vi "RF Paths Calibration Tool.vi"() -> ()   [LabVIEW 2015]
uses:
  <instrlib>/niRFSG/niRFSG.llb/niRFSG Ref Clock Sources.ctl
  <vilib>/Utility/file.llb/Read From Spreadsheet File (DBL).vi
  <vilib>/Utility/file.llb/Write To Spreadsheet File (DBL).vi
panel:
  out "Frequency (Hz)":dbl format="%.3p"
  out "Corrected Pwr (dBm)":dbl format="%.3g"
  in  "SG_Type":enum32{"ESG/PSG", "RFSG"}(tab)
  in  "Power Level Ref-ESG(dBm)":dbl caption="Power Level (dBm)" format="%.2f"
  in  "ALC":bool=TRUE
  in  "ALC BW":bool=TRUE
  in  "Pwr Srch":bool
  in  "Freq Mode":bool=TRUE
  in  "SigGen (ESG)":refnum<visa-resource-name>
  in  "Power Level - RFSG(dBm)":dbl caption="Power Level (dBm)" format="%.2f"
  in  "SigGen (RFSG)":refnum<k15>
  in  "Loop Delay(ms)":i32=100
  in  "Secure Display":bool
  in  "Config Save":bool
  in  "Start":bool
  in  "Stop":bool
  in  "Help":bool
  out "main_queue":refnum<user-event>
  in  "Export Plots to Excel?":bool
  in  "PM Type":T1(tab)=enum."U2000 USB [PM2]"
  in  "Measuring Function":i32(ring) items=["Single", "Single Relative", "Difference", "Difference Relative", "Ratio", "Ratio Relative"]
  in  "Channel":i32(ring) items=["A", "B"]
  in  "Resolution":i32=3
  in  "Avg Count":i32=3
  in  "PM State":bool
  in  "Measurement Speed":i32(ring)=2 items=["Normal", "Double", "Fast"]
  in  "Sensor 1 Channel":i32(ring) items=["Channel A", "Channel B"]
  in  "Sensor 2 Channel":i32(ring) items=["Channel A", "Channel B"]
  in  "Auto Clear":i32(ring) items=["Off", "On", "ONCE"]
  in  "EPM GPIB ALIAS":refnum<visa-resource-name>
  in  "Units":i32(ring) items=["dBm", "W"]
  in  "Trigger Level (dBm)":dbl
  in  "Averaging Count":i32=3 min=1 max=100 step=1
  in  "Trigger Source":i32(ring)=3 items=["Bus", "External", "Hold", "Immediate", "Internal A"]
  in  "Trigger Slope":u16(ring) items=["Positive", "Negative"]
  in  "Enable Averaging":bool
  in  "U2000 GPIB ALIAS":refnum<visa-resource-name>
  in  "Atten (dB)":dbl=20.0
  in  "Auto Atten":bool
  in  "Averaging":bool=TRUE
  in  "Auto Align":bool=TRUE
  in  "Zero Span":bool=TRUE
  in  "Avg":i32=10
  in  "Ref Lvl (dBm)":dbl=10.0 min=-100.0 max=30.0 step=0.1
  in  "SpecAn Mode":enum32{"Manual", "Auto"}(tab)
  in  "VBW (Hz)":i32=300000 format="%.0p"
  in  "RBW (Hz)":i32=100000 format="%.0p"
  in  "Span (Hz)":dbl=100000.0 format="%#_13p"
  in  "PSA E4440A GPIB":refnum<visa-resource-name>
  out "Status":string
  out "Path Loss":cluster{dbl[]}[](graph)
  in  "Tab Control":enum32{"Arbitrary", "Lookup Table"}(tab)=enum."Lookup Table"
  in  "Intervals (Hz)":dbl=1000000.0 min=100000.0 max=1000000000.0 step=100000.0 format="%.3p"
  in  "Stop F (Hz)":dbl=6000000000.0 min=1000000.0 max=18000000000.0 step=1000000.0 format="%.3p"
  in  "Start F (Hz)":dbl=10000000.0 min=1000000.0 max=18000000000.0 step=1000000.0 format="%.3p"
  in  "file path (dialog if empty)":path
  out "Normalization Active":bool
  in  "Normalization Files":path[](array[path])
  out "Error Out":errorcluster {"code" format="%.0x"}
  # "rev: 3.0.1"
  # "CW/Signal Generator Configuration"
  # "CW"
  # "FIX"
  # "RBW/VBW Settings\nNot  Required"
  # "Measuring Device Configuration [Select Type]"
  # "Frequency Sweep Parameters"
  # "RF Paths Calibration Tool"
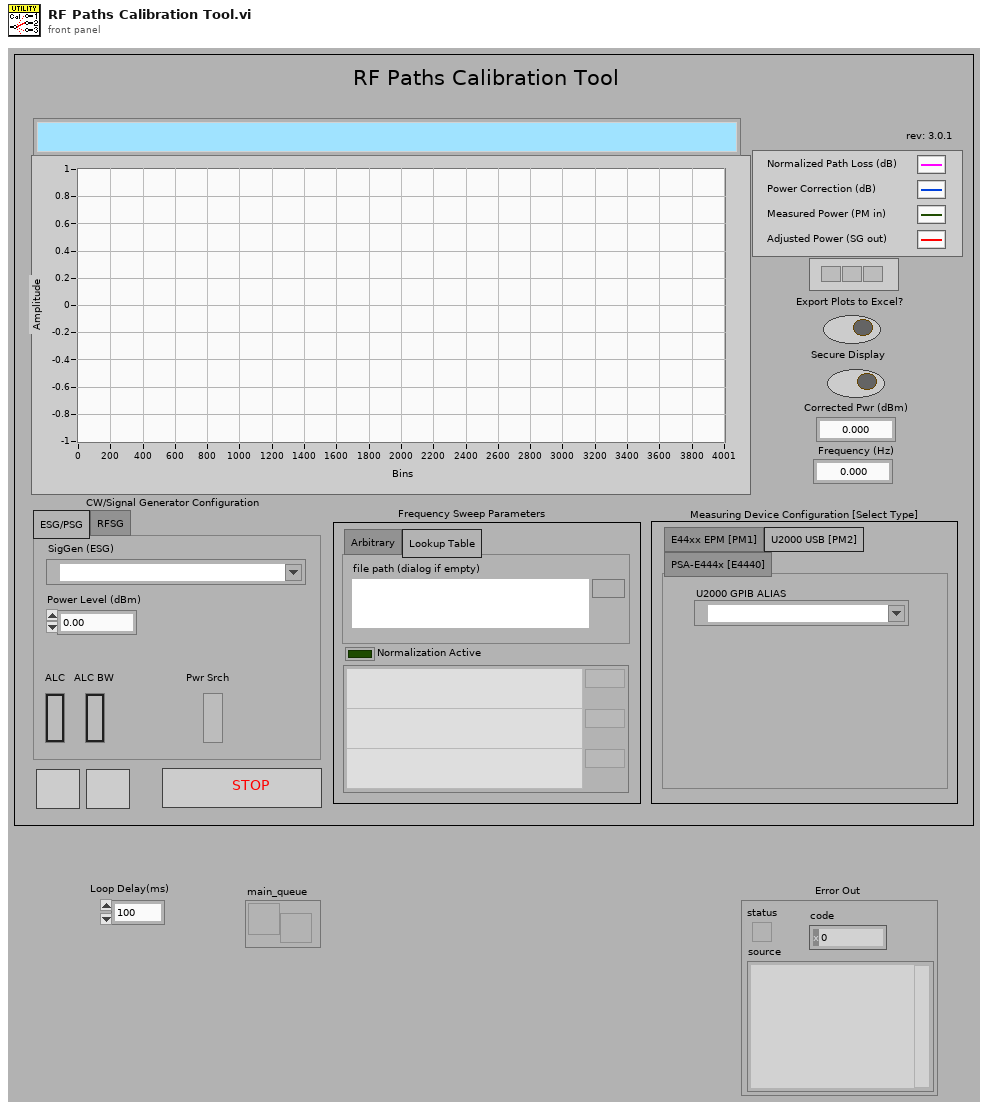
[diagram p1: front panel]
types:
  T1 = enum32{"E44xx EPM [PM1]", "U2000 USB [PM2]", "PSA-E444x [E4440]"}
  T2 = enum32{"invalid app kind", "Development System", "Run Time System", "Student Edition", "Embedded LabVIEW", "Evaluation", "Custom"}
  T3 = enum32{"Invalid", "Standard", "Closed", "Hidden", "Minimized", "Maximized"}
  T4 = typedef "niRFSG Ref Clock Sources.ctl" = string
  T5 = cluster{"INI Path":path, "PSA E4440A GPIB":refnum<visa-resource-name>, "EPM GPIB ALIAS":refnum<visa-resource-name>, "U2000 GPIB ALIAS":refnum<visa-resource-name>, "SigGen (ESG)":refnum<visa-resource-name>, "SigGen (RFSG)":refnum<k15>, "Power Level Ref-ESG(dBm)":dbl, "Power Level - RFSG(dBm)":dbl, "Initial Cal Freq":dbl, "Span (Hz)":dbl, "Cal Freqs":dbl[], "Input Path Loss":dbl[], "ALC":bool, "PM State":bool, "Freq Mode":bool, "Zero Span":bool, "SG_Type":enum32{"ESG/PSG", "RFSG"}, "PM Type":enum32{"E44xx EPM [PM1]", "U2000 USB [PM2]", "PSA-E444x [E4440]"}, "Channel":i32, "Avg Count":i32, "Measurement Speed":i32, "Measuring Function":i32, "Sensor 1 Channel":i32, "Sensor 2 Channel":i32, "Unit (0: dBm)":i32, "Rows":i32, "Normalization Files":path[], "Path Loss":cluster{dbl[]}[], "Input parameters":cluster{"Channel (1)":i32, "Avg Count":i32, "Correction Frequency":dbl, "Timeout":i32, "Reset Device":bool, "ID Query":bool, "Resource Name":string, "Ref Level (dB)":dbl}, "Status":string}
  T6 = cluster{"Core":cluster{"Current VI Reference":refnum<vi>, "Close Panel on Exit?":bool}, "Your Boolean data":bool, "Your string data":string}
  T7 = cluster{"Current VI Reference":refnum<vi>, "Close Panel on Exit?":bool}
  T8 = cluster{"Channel (1)":i32, "Avg Count":i32, "Correction Frequency":dbl, "Timeout":i32, "Reset Device":bool, "ID Query":bool, "Resource Name":string, "Ref Level (dB)":dbl}
  T9 = enum8{"Enabled", "Disabled", "Disabled and Grayed Out"}
  T10 = enum16{"Left Button", "Center Button", "Right Button", "Window Close"}
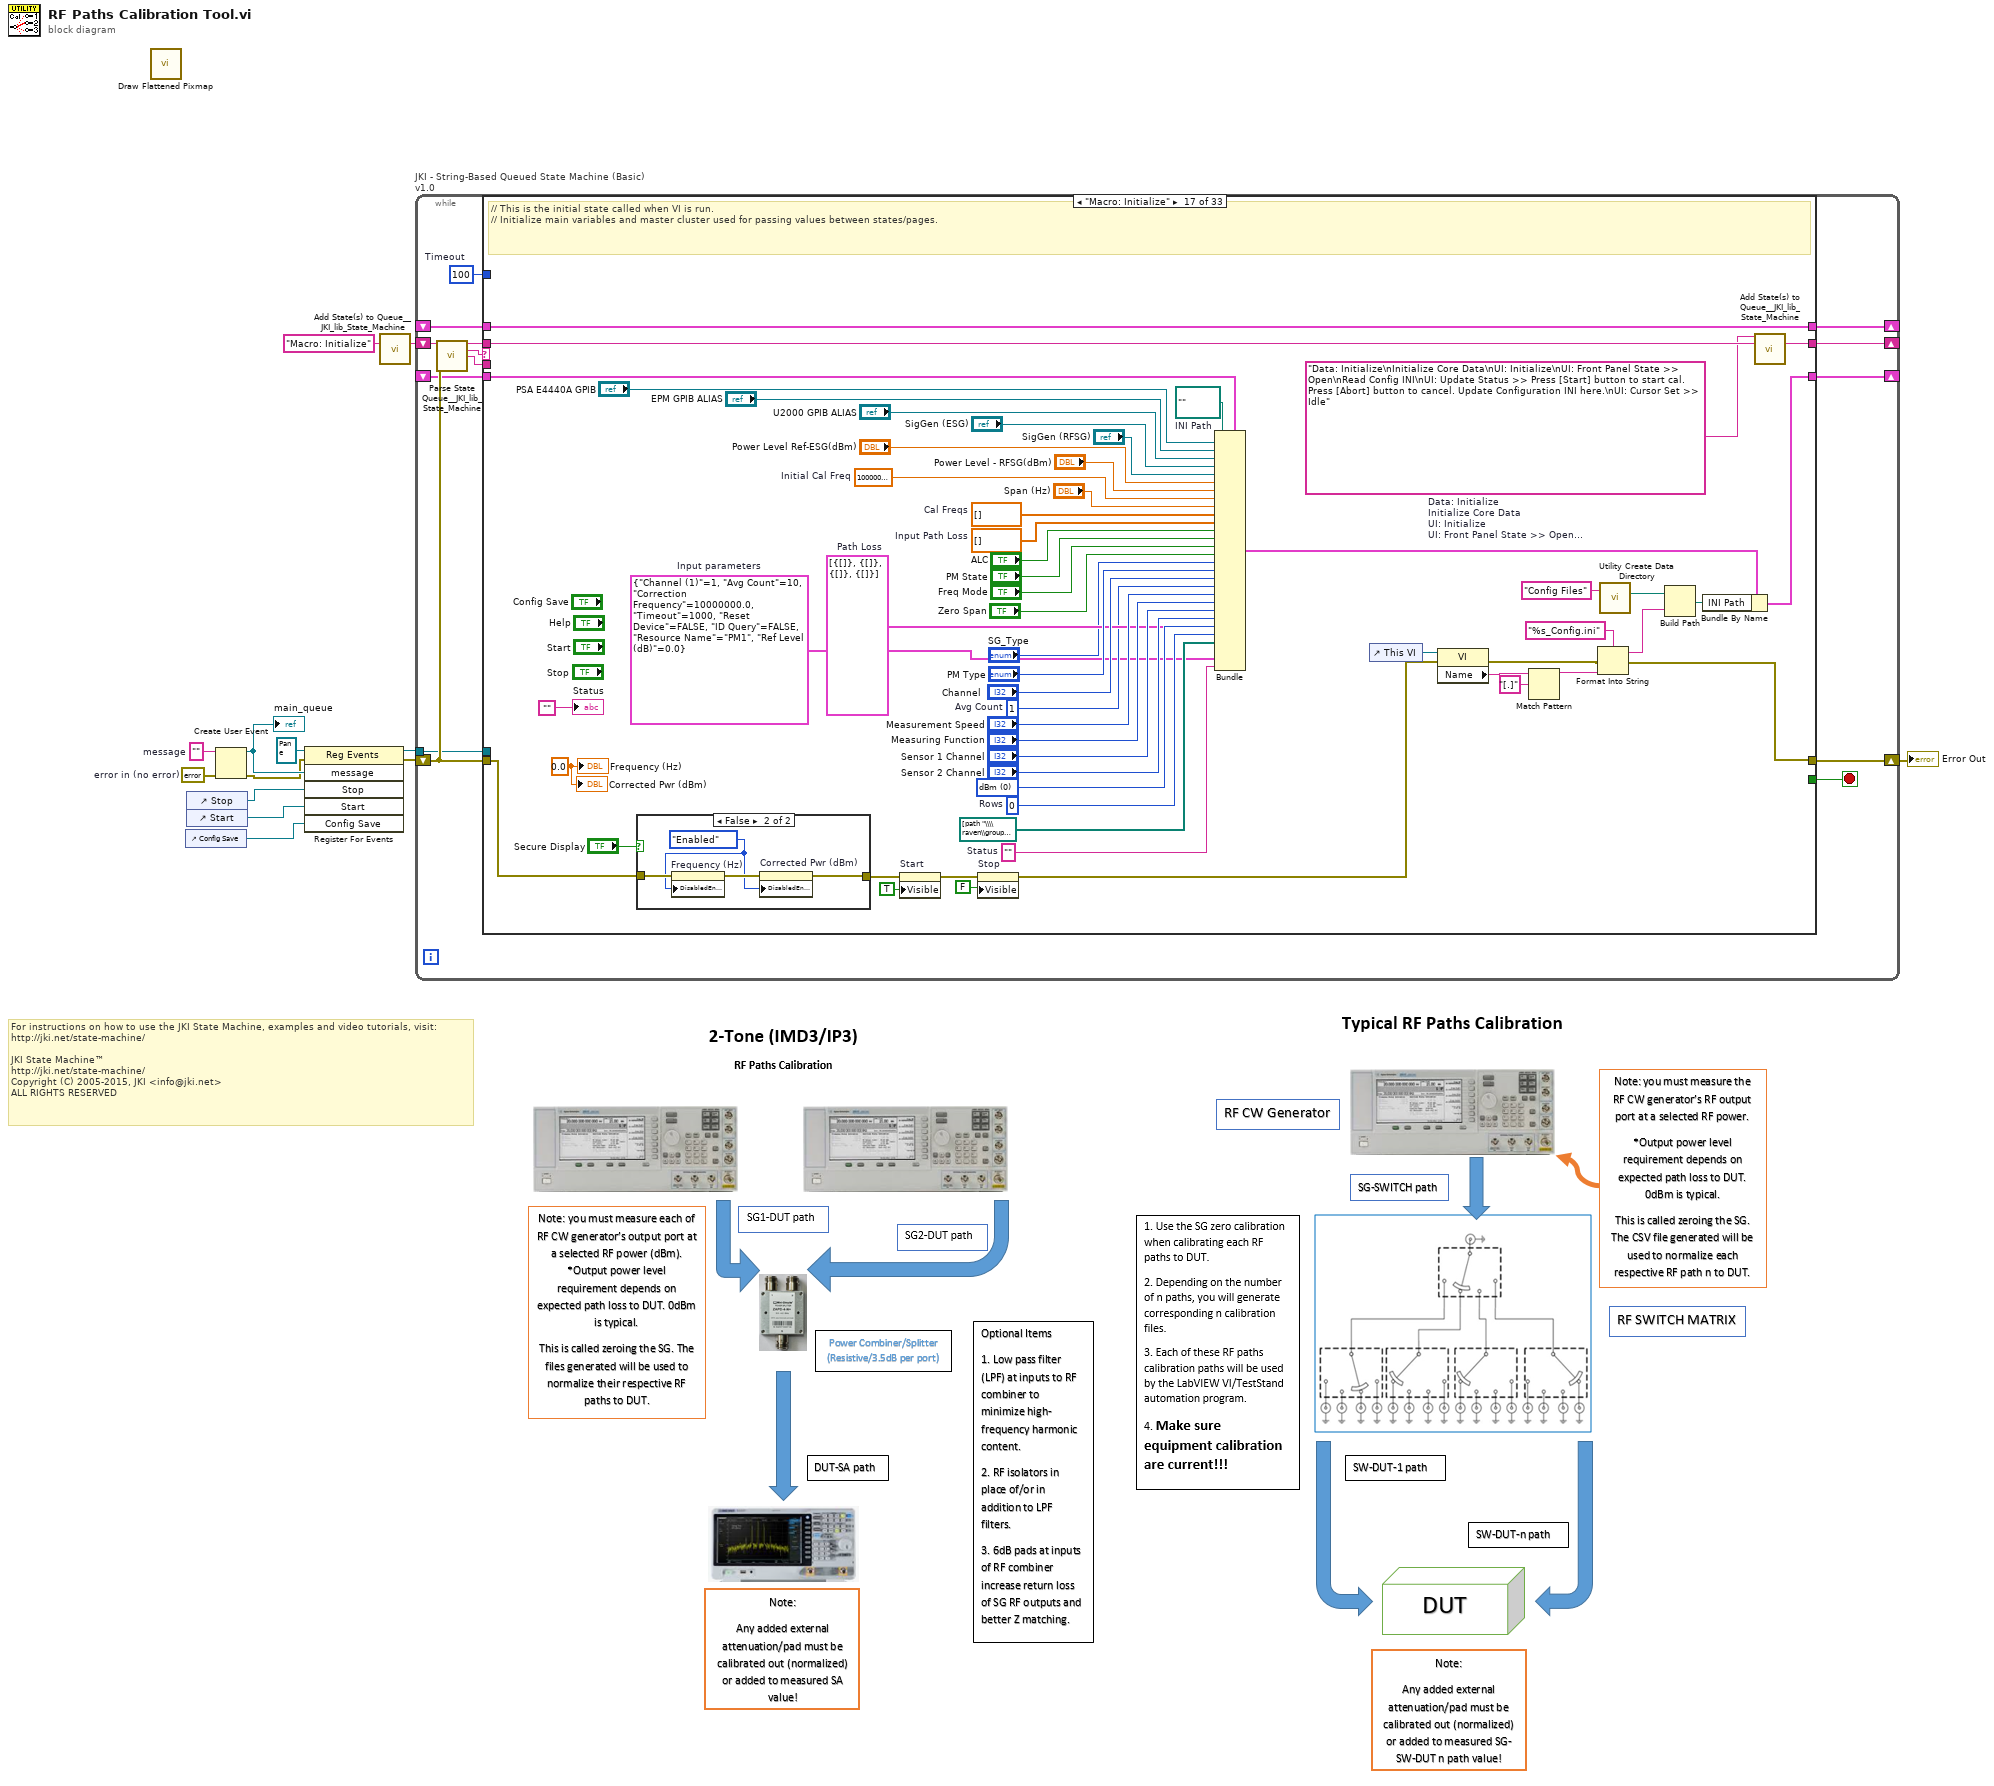
[diagram p0: block diagram]
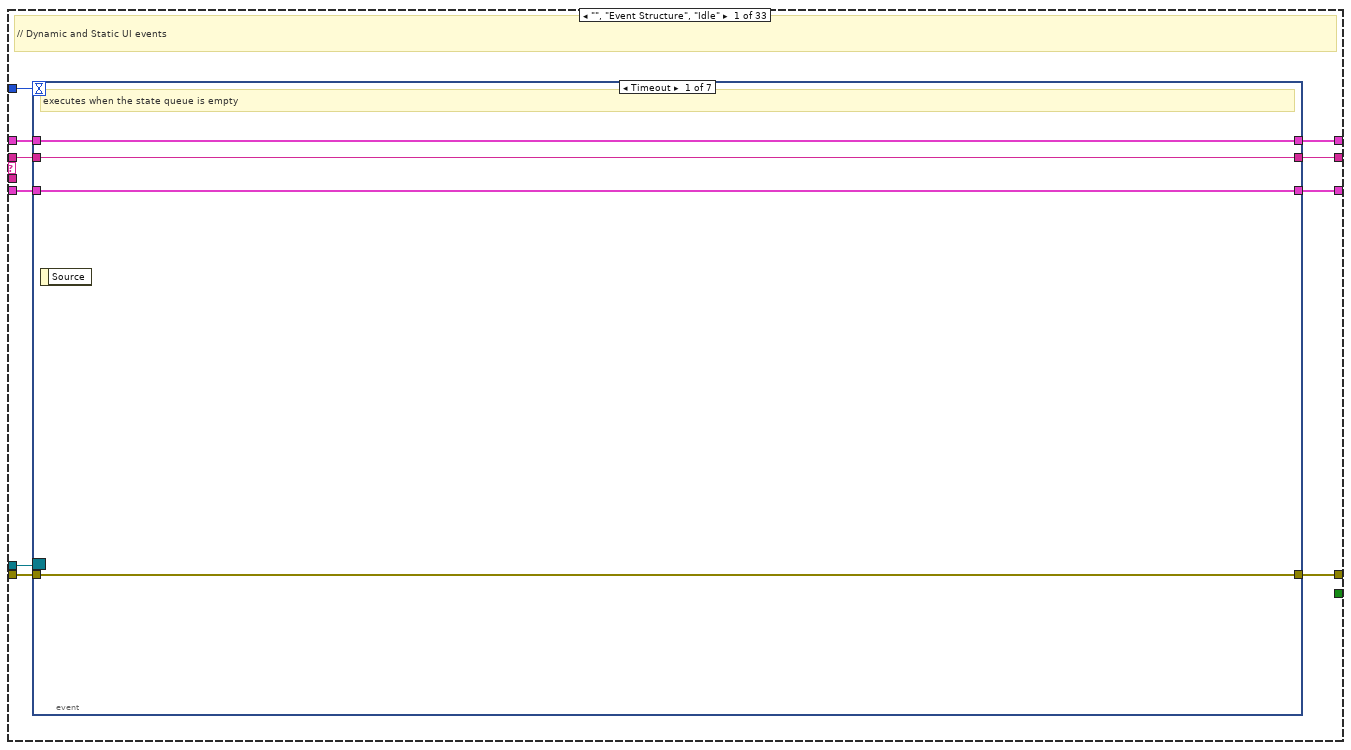
[diagram p2: hidden frame]
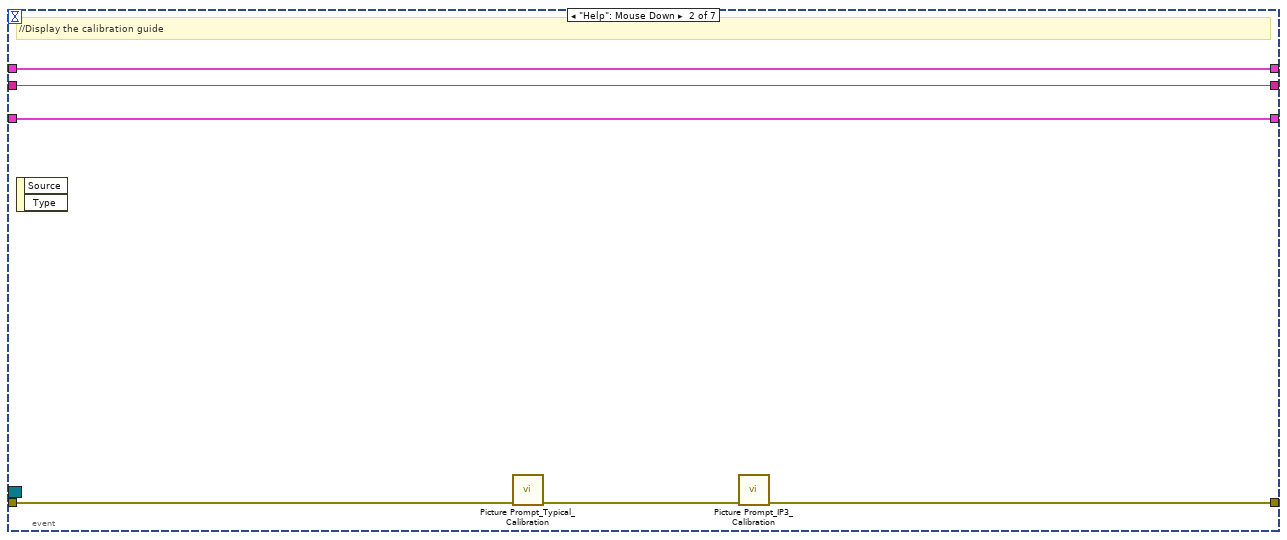
[diagram p3: hidden frame]
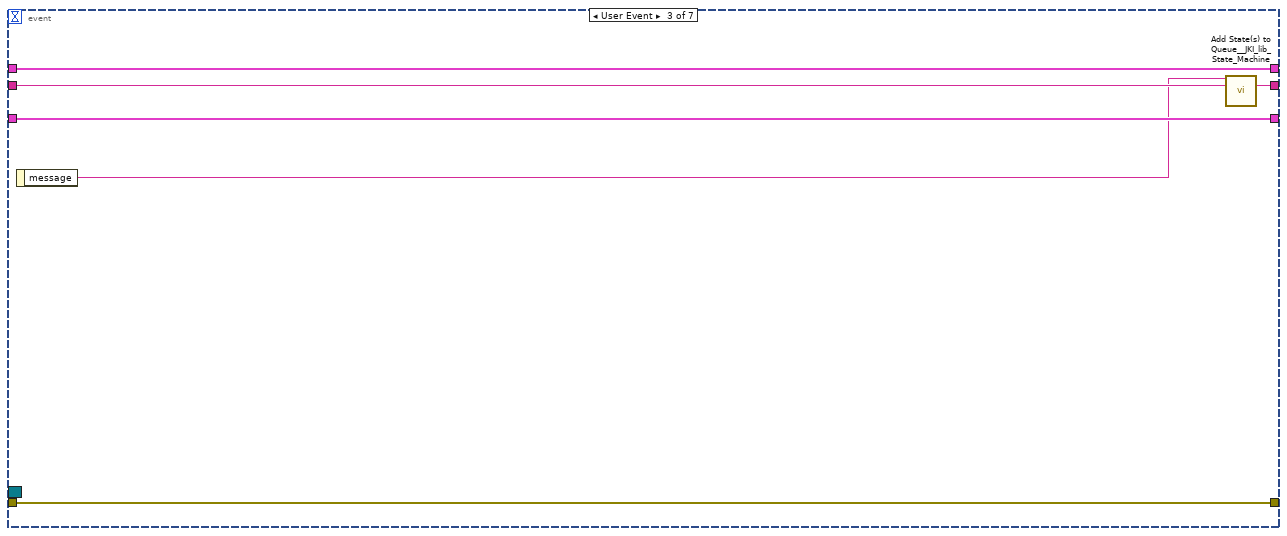
[diagram p4: hidden frame]
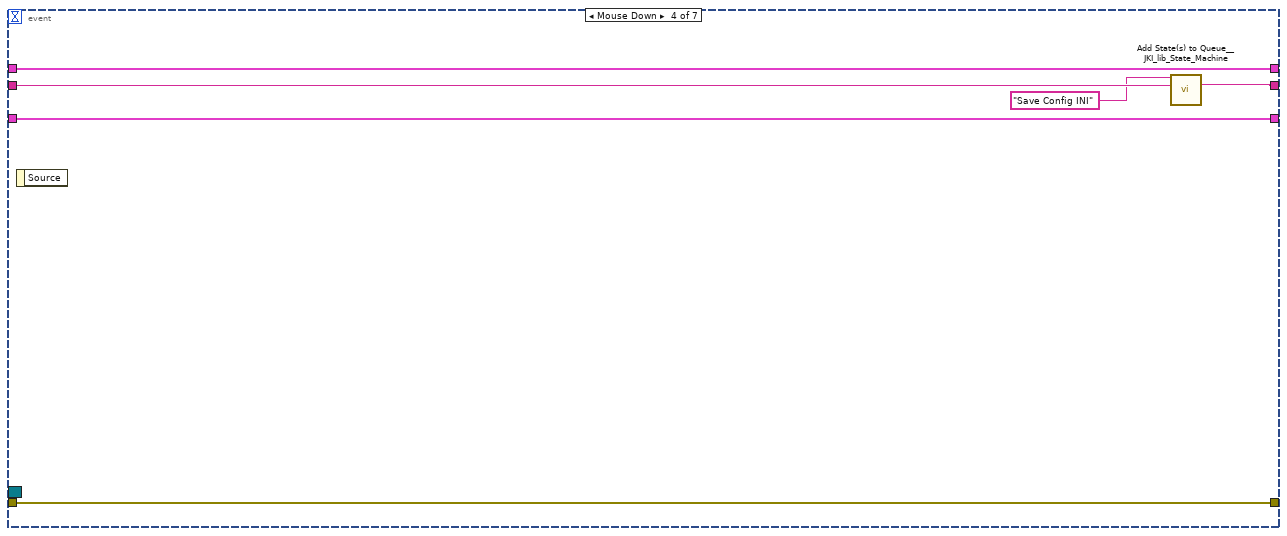
[diagram p5: hidden frame]
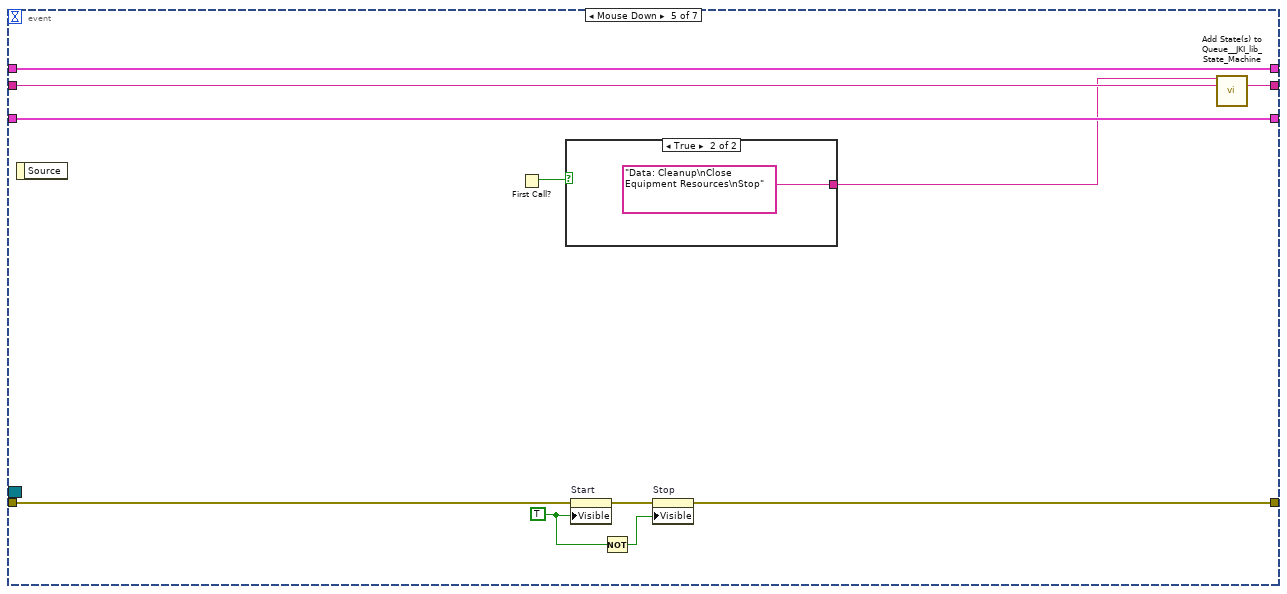
[diagram p6: hidden frame]
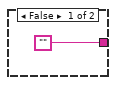
[diagram p7: hidden frame]
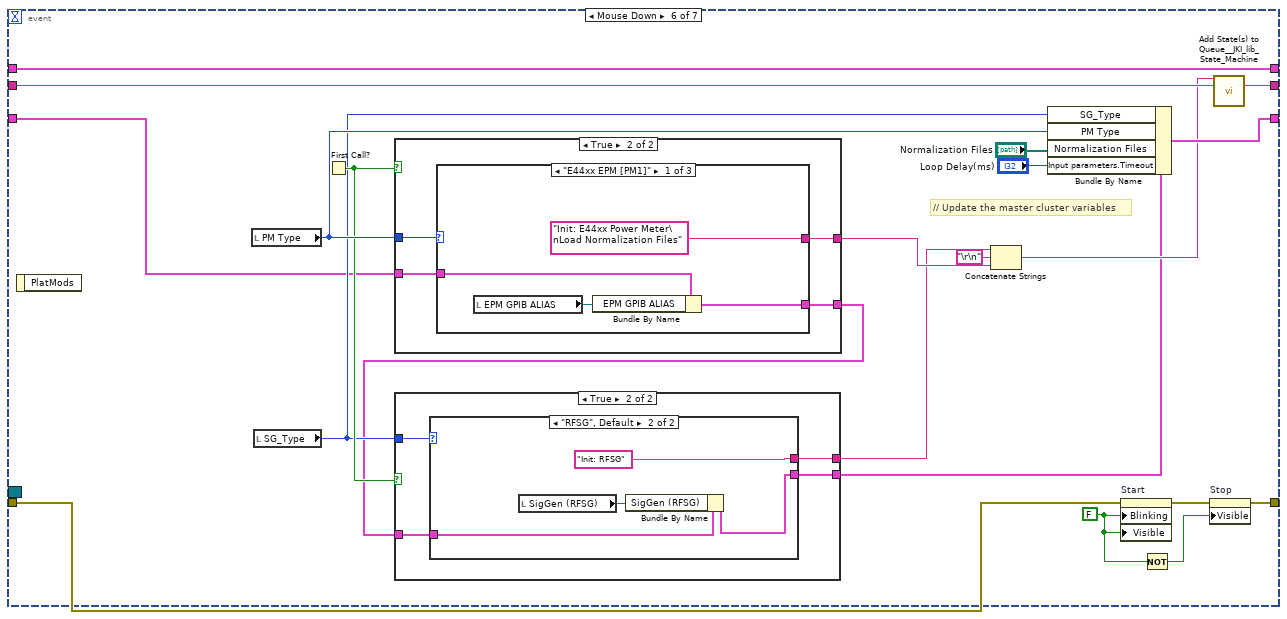
[diagram p8: hidden frame]
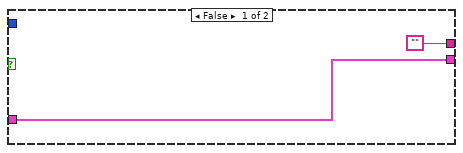
[diagram p9: hidden frame]
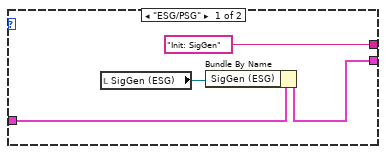
[diagram p10: hidden frame]
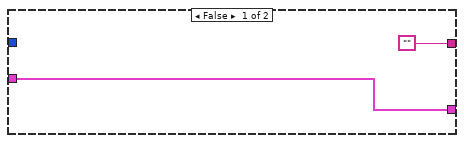
[diagram p11: hidden frame]
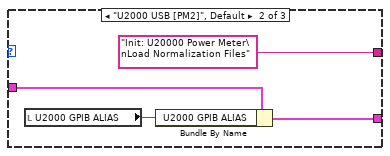
[diagram p12: hidden frame]
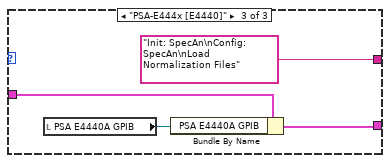
[diagram p13: hidden frame]
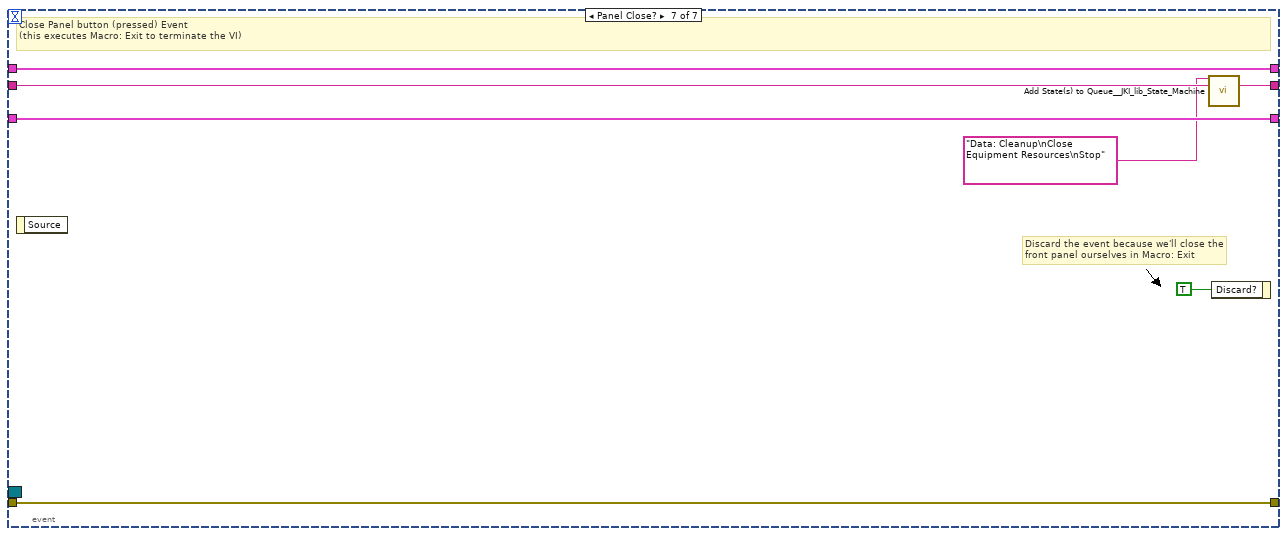
[diagram p14: hidden frame]
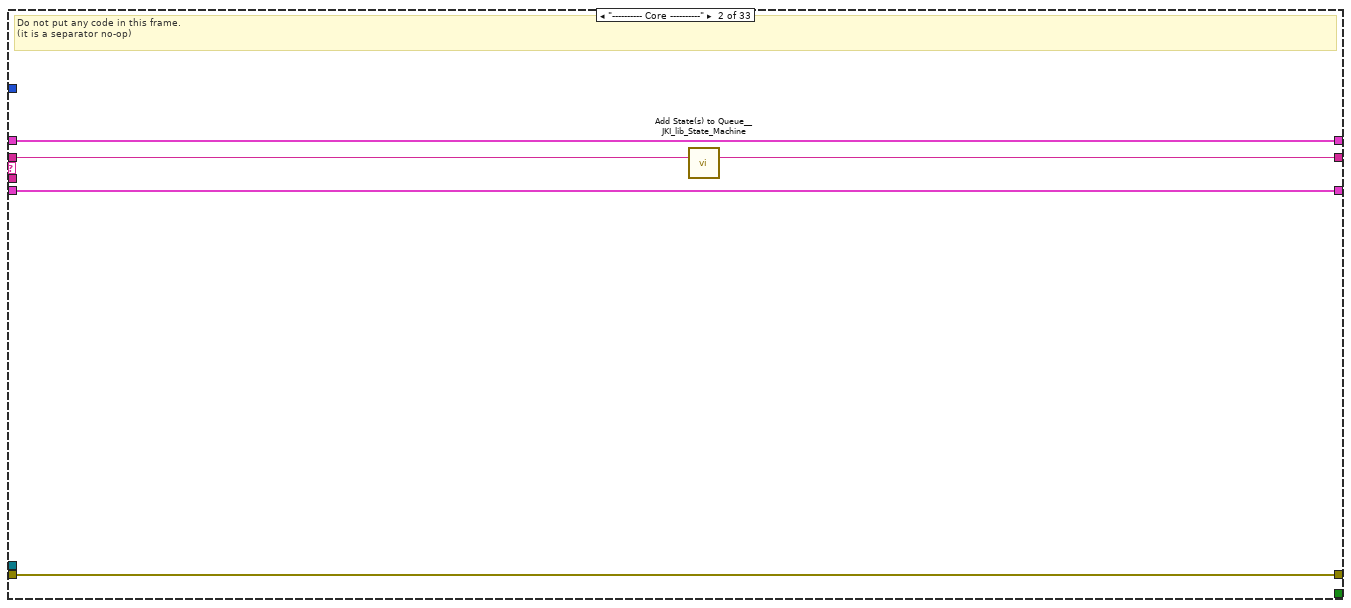
[diagram p15: hidden frame]
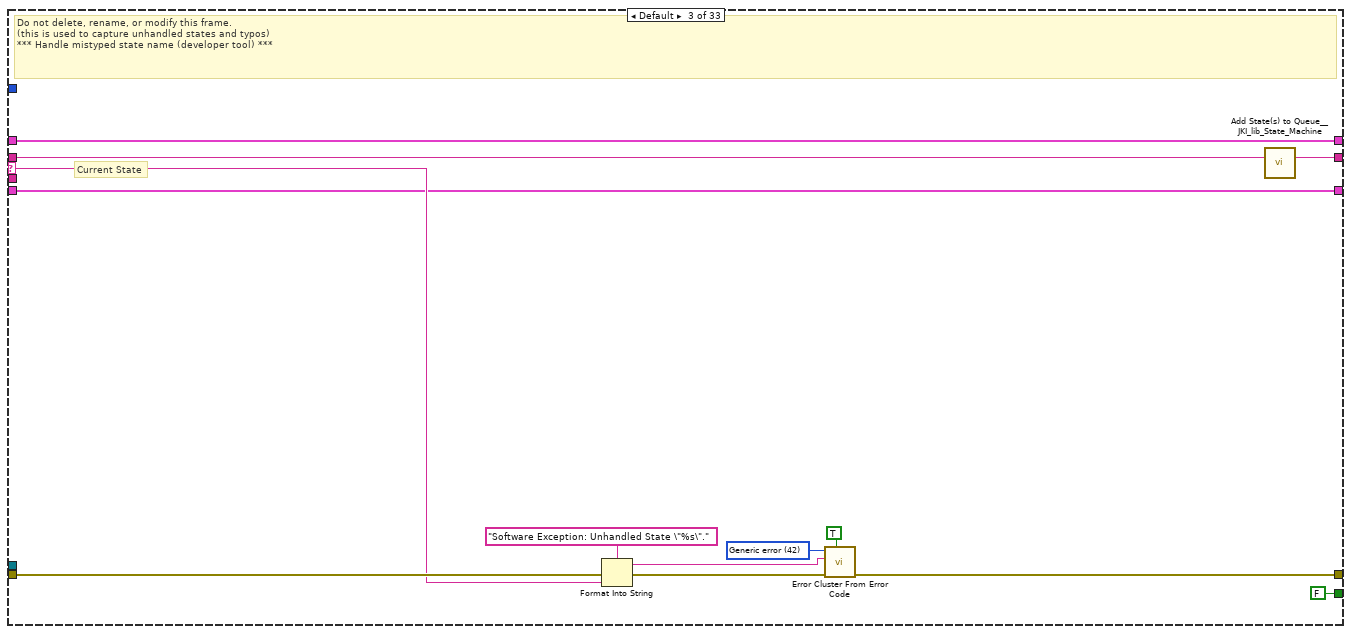
[diagram p16: hidden frame]
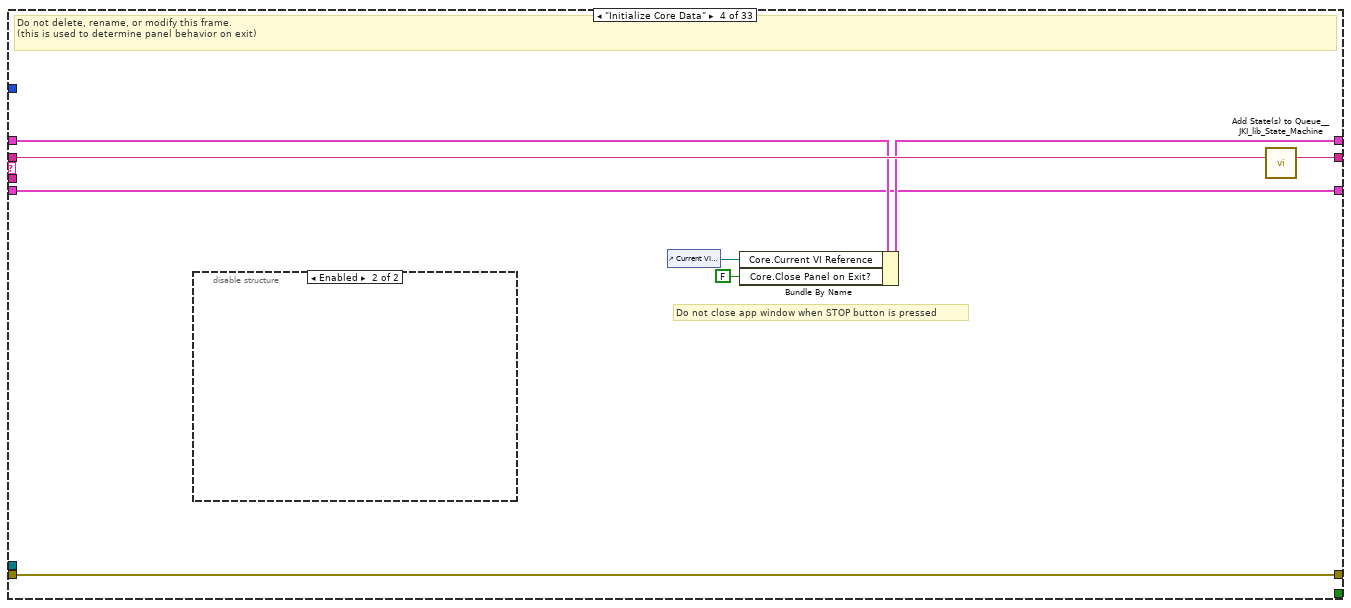
[diagram p17: hidden frame]
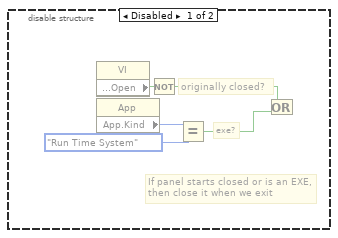
[diagram p18: hidden frame]
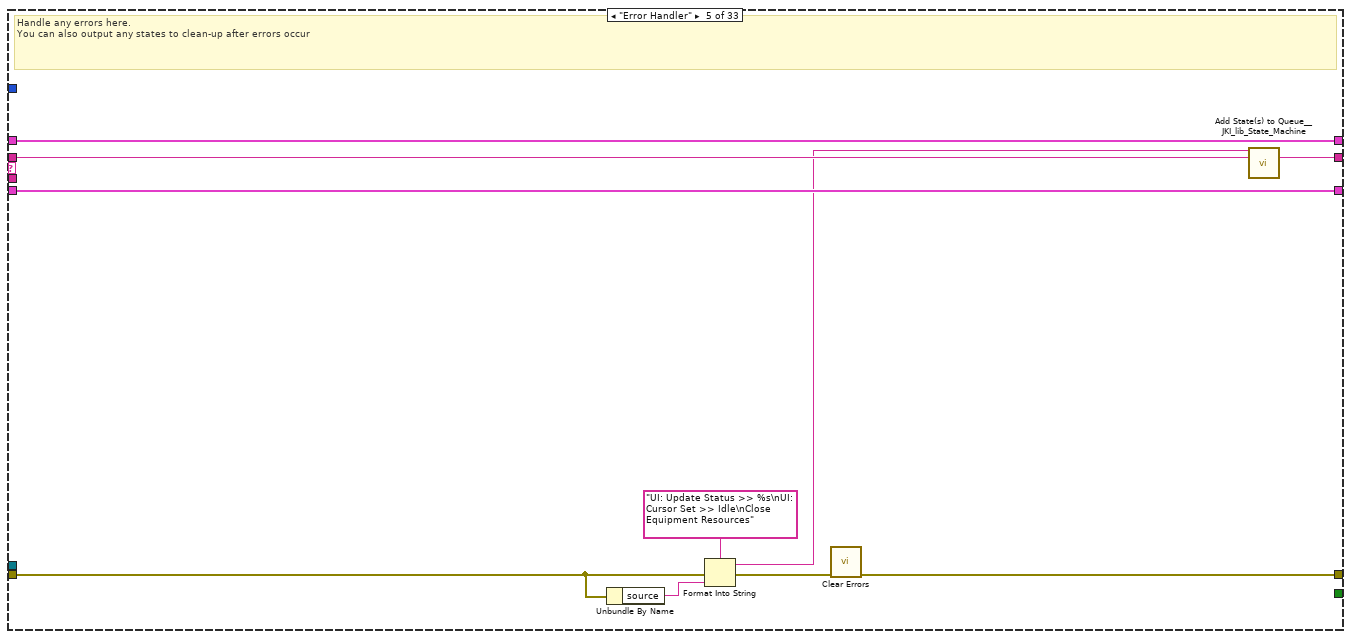
[diagram p19: hidden frame]
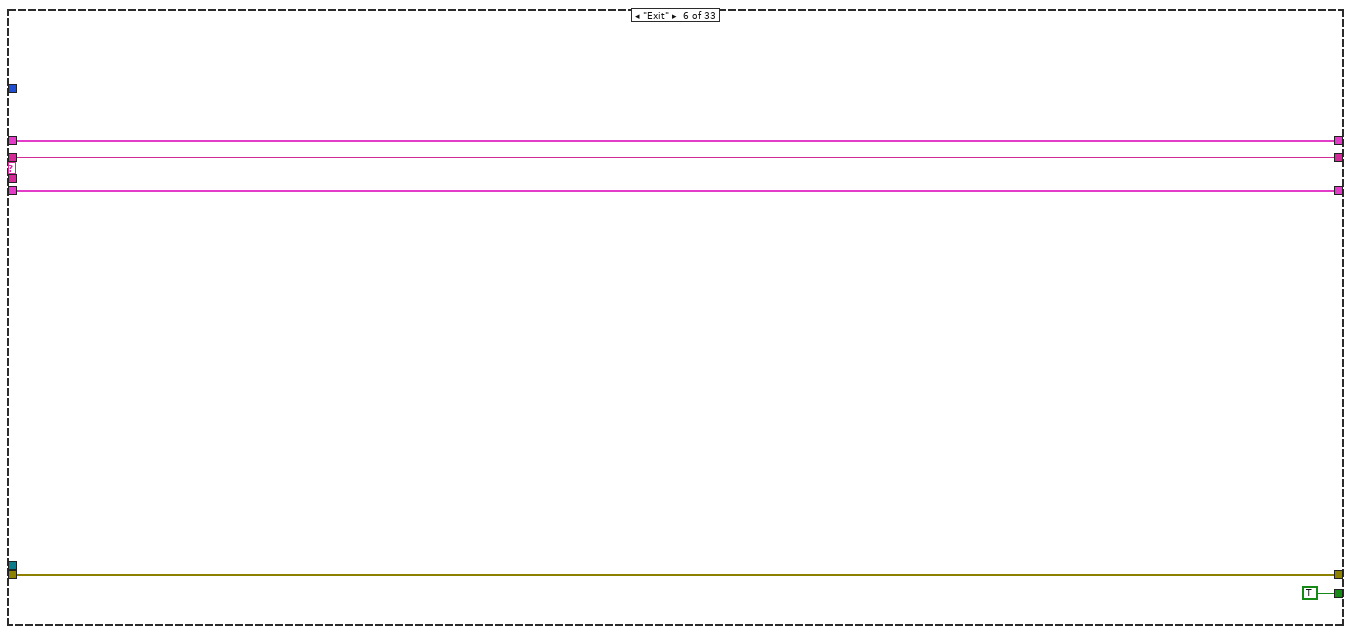
[diagram p20: hidden frame]
diagram:
  w10 = ""  # message
  w9 = errorcluster {"status"=FALSE, "code"=0, "source"=""}  # error in (no error)
  # "For instructions on how to use the JKI State Machine, examples and video tutorials, visit:\nhttp://jki.net/state-machine/\n\nJKI State Machine™\nhttp://jki.net/state-machine/\nCopyright (C) 2005-2015, JKI <info@jki.net>\nALL RIGHTS RESERVED"
  n1 = call <vilib>:"Draw Flattened Pixmap.vi"() -> ()  [unwired: 9 in, 1 out]
  n2 = control-ref of="Config Save"() -> (w4:refnum<vi>)
  n3 = control-ref of="Stop"() -> (w2:refnum<vi>)
  n4 = control-ref of="Start"() -> (w3:refnum<vi>)
  n5 = Create User Event(user event datatype=w10, error in=w9) -> (user event=w8:refnum<user-event>, error out=w7:errorcluster)
  "main_queue" <- w8
  n6 = register-events(reference=refnum<event-registration> refnum ("event registration refnum"), error in=w7, w8, w2, w3, w4) -> (reference out=w5:refnum<event-registration>, error out=w6:errorcluster)
  n7 = call <vilib>:"Add State(s) to Queue__JKI_lib_State_Machine.vi"("State(s) in (\"\")"="Macro: Initialize") -> ("States Out"=w13:string)  [unwired: 14 in]
  n8 = while "JKI - String-Based Queued State Machine (Basic) v1.0" {
    shift-right: [w21] -> _
    shift-left: _ -> [w20]
    shift-right: [w15] -> w11
    shift-left: w6 -> [w18]
    shift-right: [w23] -> _
    shift-left: w13 -> [w24]
    shift-right: [w17] -> _
    shift-left: _ -> [w16]
    tunnel: w5 -> [w14]
    stop <- w22 stop-if-true
    w19 = 100  # Timeout
    n9 = call <vilib>:"Parse State Queue__JKI_lib_State_Machine.vi"("State Queue"=w24, "Error In (no error)"=w18) -> ("Remaining States"=w26:string, "Current State"=w27:string, "Arguments"=w25:string)  [unwired: 11 in]
    n10 = case shown="\"Macro: Initialize\"" w27 {
      selector: w27 -> [_ _ w140 _ _ _ _ _ _ _ _ _ _ _ _ _ _ _ w345 w403 w456 w498 w566 w640 _ _ _ _ w728 w745 w807 w957 _]
      tunnel: w26 -> [w37 w137 w144 w158 w173 w174 w179 w188 w196 w203 w208 w213 w220 w232 w255 w264 w321 w340 w344 w417 w459 w497 w586 w650 w692 w705 w720 w721 w734 w767 w824 w963 w998]
      tunnel: w25 -> [_ _ _ _ _ _ _ _ _ _ _ _ w215 w226 w256 _ _ _ _ _ _ _ _ _ _ _ _ _ _ _ _ _ _]
      tunnel: w20 -> [w35 w134 w142 w154 w171 w178 w183 w185 _ w198 w205 w211 w218 w228 w258 w261 w319 w337 w353 w415 w470 w525 w584 w648 w689 w703 w718 w726 w732 w765 w833 w969 w1006]
      tunnel: [w34 w135 w146 w155 w168 w177 w182 w186 w193 w199 w206 w210 w216 w229 w259 w262 w272 w338 w346 w401 w453 w499 w576 w646 w690 w699 w715 w722 w730 w747 w820 w964 w1003] -> w15
      tunnel: w18 -> [w33 w135 w145 w155 w167 w177 w182 w186 w193 w200 w206 w210 w217 w230 w259 w262 w291 w338 w351 w414 w465 w528 w554 w644 w690 w700 w713 w723 w731 w755 w805 w968 w1007]
      tunnel: [w36 w136 w143 w157 w172 w174 w179 w187 w195 w202 w207 w212 w219 w231 w255 w263 w320 w339 w354 w416 w458 w496 w585 w649 w691 w704 w719 w721 w733 w766 w823 w962 w998] -> w23
      tunnel: [_ _ FALSE _ _ TRUE w180 _ _ _ _ _ _ _ _ _ _ _ _ _ _ _ _ _ _ _ _ _ _ _ _ _ _] -> w22
      tunnel: [w32 w134 w142 w156 w171 w178 w183 w185 w194 w198 w205 w211 w218 w228 w258 w261 w319 w337 w353 w415 w470 w525 w584 w648 w689 w703 w718 w726 w732 w765 w833 w969 w1006] -> w21
      tunnel: w19 -> [w31 _ _ _ _ _ _ _ _ _ _ _ _ _ _ _ _ _ _ _ _ _ _ _ _ _ _ _ _ _ _ _ _]
      tunnel: [w29 w133 w138 w152 w170 w175 w181 w184 w189 w197 w204 w209 w214 w225 w257 w260 w274 w330 w342 w413 w467 w502 w565 w639 w688 w698 w709 w725 w727 w752 w828 w960 w1005] -> w17
      tunnel: w16 -> [w30 w133 w138 w152 w170 w175 w181 w184 w189 w197 w204 w209 w214 w225 w257 w260 w316 w330 w352 w413 w467 w502 w581 w647 w688 w698 w709 w725 w727 w753 w832 w960 w1005]
      tunnel: w14 -> [w28 _ _ _ _ _ _ _ _ _ _ _ _ _ _ _ _ _ _ _ _ _ _ _ _ _ _ _ _ _ _ _ _]
      frame "", "Event Structure", "Idle" {
        # "// Dynamic and Static UI events"
        n11 = event shown="[0] Timeout" {
          selector: w28 -> [_ _ _ _ _ _ _]
          dyn-events: _ -> [_ _ _ _ _ _ _]
          timeout: w31 -> [_ _ _ _ _ _ _]
          tunnel: w37 -> [w38 w42 w50 w57 w67 w92 w132]
          tunnel: [w38 w42 w49 w56 w66 w91 w131] -> w36
          tunnel: w35 -> [w40 w46 w52 w58 w68 w93 w129]
          tunnel: [w41 w43 w51 w55 w63 w89 w130] -> w34
          tunnel: w33 -> [w41 w45 w51 w55 w64 w73 w130]
          tunnel: [w40 w46 w52 w58 w68 w93 w129] -> w32
          tunnel: w30 -> [w39 w47 w53 w59 w70 w76 w127]
          tunnel: [w39 w47 w53 w59 w70 w85 w127] -> w29
          event Timeout {
            # "executes when the state queue is empty"
            n12 = event-data() -> ()  [unwired: 1 in, 1 out]
          }
          event "Help": Mouse Down {
            # "//Display the calibration guide"
            n13 = event-data() -> ()  [unwired: 1 in, 2 out]
            n14 = call "Picture Prompt_Typical_Calibration.vi"("error in (no error)"=w45) -> ("error out"=w44:errorcluster)  [unwired: 9 in, 1 out]
            n15 = call "Picture Prompt_IP3_Calibration.vi"("error in (no error)"=w44) -> ("error out"=w43:errorcluster)  [unwired: 9 in, 1 out]
          }
          event User Event {
            n16 = event-data() -> ("message"=w48:string)  [unwired: 1 in]
            n17 = call <vilib>:"Add State(s) to Queue__JKI_lib_State_Machine.vi"("State(s) in Front (\"\")"=w48, "State(s) in (\"\")"=w50) -> ("States Out"=w49:string)  [unwired: 13 in]
          }
          event Mouse Down {
            n18 = event-data() -> ()  [unwired: 1 in, 1 out]
            n19 = call <vilib>:"Add State(s) to Queue__JKI_lib_State_Machine.vi"("State(s) in Front (\"\")"="Save Config INI" ("State(s) in Front (\"\")"), "State(s) in (\"\")"=w57) -> ("States Out"=w56:string)  [unwired: 13 in]
          }
          event Mouse Down {
            w61 = TRUE ("Visible")
            n20 = event-data() -> ()  [unwired: 1 in, 1 out]
            n21 = First Call?() -> (First Call?: T/F=w69:bool)
            n22 = case shown="True" w69 {
              tunnel: ["" "Data: Cleanup\nClose Equipment Resources\nStop"] -> w65
              frame False {
              }
              frame True {
              }
            }
            n23 = property on="Start" class="Bool (strict)"(error in=w64, "Visible"=w61) -> (error out=w62:errorcluster)  [unwired: 1 in, 1 out]
            n24 = Not(x=w61) -> (.not. x?=w60:bool)
            n25 = property on="Stop" class="Bool (strict)"(error in=w62, "Visible"=w60) -> (error out=w63:errorcluster)  [unwired: 1 in, 1 out]
            n26 = call <vilib>:"Add State(s) to Queue__JKI_lib_State_Machine.vi"("State(s) in Front (\"\")"=w65, "State(s) in (\"\")"=w67) -> ("States Out"=w66:string)  [unwired: 13 in]
          }
          event Mouse Down {
            w87 = FALSE ("Blinking")
            # "// Update the master cluster variables"
            n27 = event-data() -> ()  [unwired: 1 in, 1 out]
            n28 = local read "PM Type"() -> (w83:T1)
            n29 = local read "SG_Type"() -> (w80:enum32{"ESG/PSG", "RFSG"})
            n30 = First Call?() -> (First Call?: T/F=w81:bool)
            n31 = case shown="True" w81 {
              tunnel: ["" w113] -> w90
              tunnel: w83 -> [_ w112]
              tunnel: w76 -> [w108 w111]
              tunnel: [w108 w110] -> w74
              frame False {
              }
              frame True {
                n32 = case shown="\"E44xx EPM [PM1]\"" w112 {
                  tunnel: ["Init: E44xx Power Meter\nLoad Normalization Files" "Init: U20000 Power Meter\nLoad Normalization Files" "Init: SpecAn\nConfig: SpecAn\nLoad Normalization Files"] -> w113
                  tunnel: w111 -> [w116 w120 w123]
                  tunnel: [w115 w119 w124] -> w110
                  frame "E44xx EPM [PM1]" {
                    n33 = local read "EPM GPIB ALIAS"() -> (w114:refnum<visa-resource-name>)
                    n34 = Bundle By Name(cluster=w116, "EPM GPIB ALIAS"=w114) -> (w115:T5)
                  }
                  frame "U2000 USB [PM2]", Default {
                    n35 = local read "U2000 GPIB ALIAS"() -> (w118:refnum<visa-resource-name>)
                    n36 = Bundle By Name(cluster=w120, "U2000 GPIB ALIAS"=w118) -> (w119:T5)
                  }
                  frame "PSA-E444x [E4440]" {
                    n37 = local read "PSA E4440A GPIB"() -> (w122:refnum<visa-resource-name>)
                    n38 = Bundle By Name(cluster=w123, "PSA E4440A GPIB"=w122) -> (w124:T5)
                  }
                }
              }
            }
            n39 = case shown="True" w81 {
              tunnel: w80 -> [_ w99]
              tunnel: ["" w98] -> w78
              tunnel: [w94 w97] -> w75
              tunnel: w74 -> [w94 w96]
              frame False {
              }
              frame True {
                n40 = case shown="\"RFSG\", Default" w99 {
                  tunnel: ["Init: SigGen" "Init: RFSG"] -> w98
                  tunnel: [w101 w105] -> w97
                  tunnel: w96 -> [w102 w106]
                  frame "ESG/PSG" {
                    n41 = local read "SigGen (ESG)"() -> (w100:refnum<visa-resource-name>)
                    n42 = Bundle By Name(cluster=w102, "SigGen (ESG)"=w100) -> (w101:T5)
                  }
                  frame "RFSG", Default {
                    n43 = local read "SigGen (RFSG)"() -> (w104:refnum<k15>)
                    n44 = Bundle By Name(cluster=w106, "SigGen (RFSG)"=w104) -> (w105:T5)
                  }
                }
              }
            }
            n45 = Concatenate Strings(w78, "\r\n", w90) -> (w79:string)
            n46 = Bundle By Name(cluster=w75, "SG_Type"=w80, "PM Type"=w83, "Normalization Files"="Normalization Files", "Input parameters.Timeout"="Loop Delay(ms)") -> (w85:T5)
            n47 = property on="Start" class="Bool (strict)"(error in=w73, "Blinking"=w87, "Visible"=w87) -> (error out=w88:errorcluster)  [unwired: 1 in, 1 out]
            n48 = Not(x=w87) -> (.not. x?=w86:bool)
            n49 = property on="Stop" class="Bool (strict)"(error in=w88, "Visible"=w86) -> (error out=w89:errorcluster)  [unwired: 1 in, 1 out]
            n50 = call <vilib>:"Add State(s) to Queue__JKI_lib_State_Machine.vi"("State(s) in Front (\"\")"=w79, "State(s) in (\"\")"=w92) -> ("States Out"=w91:string)  [unwired: 13 in]
          }
          event Panel Close? {
            # "Discard the event because we'll close the front panel ourselves in Macro: Exit"
            # "Close Panel button (pressed) Event\n(this executes Macro: Exit to terminate the VI)"
            n51 = event-data() -> ()  [unwired: 1 in, 1 out]
            n52 = call <vilib>:"Add State(s) to Queue__JKI_lib_State_Machine.vi"("State(s) in Front (\"\")"="Data: Cleanup\nClose Equipment Resources\nStop", "State(s) in (\"\")"=w132) -> ("States Out"=w131:string)  [unwired: 13 in]
            n53 = event-data("Discard?"=TRUE) -> ()  [unwired: 1 in, 1 out]
          }
        }
      }
      frame "---------- Core ----------" {
        # "Do not put any code in this frame.\n(it is a separator no-op)"
        n54 = call <vilib>:"Add State(s) to Queue__JKI_lib_State_Machine.vi"("State(s) in (\"\")"=w137) -> ("States Out"=w136:string)  [unwired: 14 in]
      }
      frame Default {
        w149 = 42 items=["No error", "Argument error", "Memory is full", "Out of zone", "End of file", "File already open", "Generic file I/O error", "File not found", "File permission error", "Disk is full", "Duplicate path", "Too many files open", "System feature not enabled", "Resource file not found", "Cannot add resource", "Resource not found", "Image not found", "Image memory error", "Pen does not exist", "Config type invalid", "Config token not found", "Config parse error", "Config memory error", "Bad external code format", "Bad external code offset", "External code not present", "Null window", "Destroy window error", "Null menu", "Print aborted", "Bad print record", "Print driver error", "Windows error during printing", "Memory error during printing", "Print dialog error", "Generic print error", "Invalid device refnum", "Device not found", "Device parameter error", "Device unit error", "Cannot open device", "Device call aborted", "Generic error", "Cancelled by user", "Object ID too low", "Object ID too high", "Object not in heap", "Unknown heap", "Unknown object (invalid DefProc)", "Unknown object (DefProc not in table)", "Message out of range", "Invalid (null) method", "Unknown message", "Manager call not supported", "Bad address", "Network operation in progress", "Network operation timed out", "Connection is busy", "Network attribute not supported", "Network error", "Address in use", "System out of memory", "Connection aborted", "Connection refused", "Not connected", "Already connected", "Connection closed", "Initialization error (interapplication manager)", "Bad occurrence", "Wait on unbound occurrence handler", "Occurrence queue overflow", "Datalog type conflict", "Unused", "Unrecognized type (interapplication manager)", "Memory corrupt", "Failed to make temporary DLL", "Old CIN version", "Drag socket not found", "Failed to load drop-object", "Failed to register OLE object", "Failed to release OLE object", "Format specifier type mismatch", "Unknown format specifier", "Too few format specifiers", "Too many format specifiers", "Scan failed", "Newer CIN version", "Error converting to variant", "Runtime menu error", "Password tampered", "Variant attribute not found", "Incompatible variant data type", "Event data is not available", "Event Store is not present", "Occurrence is not found", "Event Queue is not created", "Event info is not available", "Refnum passed is NULL", "Error retrieving Class GUID", "Error retrieving CoClass GUID", "Error retrieving TypeLib GUID.", "Bad built application magic bytes.", "Specific driver is different from the specific driver associated with the Logical Name.", "There is no session opened to the class driver.", "Max Error", "MAX - Error with config objects", "MAX - Error loading configuration", "MAX - Group not supported"]
        # "Current State"
        # "Do not delete, rename, or modify this frame.\n(this is used to capture unhandled states and typos)\n*** Handle mistyped state name (developer tool) ***"
        n55 = Format Into String(format string="Software Exception: Unhandled State \"%s\"." ("message"), error in=w145, w140) -> (resulting string=w148:string, error out=w147:errorcluster)  [unwired: 1 in]
        n56 = call <vilib>:"Error Cluster From Error Code.vi"("show call chain? (False)"=TRUE, "error in (no error)"=w147, "error message (\"\")"=w148, "error code (0)"=w149) -> ("error out"=w146:errorcluster)  [unwired: 5 in]
        n57 = call <vilib>:"Add State(s) to Queue__JKI_lib_State_Machine.vi"("State(s) in (\"\")"=w144) -> ("States Out"=w143:string)  [unwired: 14 in]
      }
      frame "Initialize Core Data" {
        # "Do not close app window when STOP button is pressed"
        # "Do not delete, rename, or modify this frame.\n(this is used to determine panel behavior on exit)"
        n58 = disable-structure shown="Enabled" {
          frame Disabled {
            # "originally closed?"
            # "exe?"
            # "If panel starts closed or is an EXE, then close it when we exit"
            n59 = property class="VI"() -> ("Front Panel.Open"=w163:bool)  [unwired: 2 in, 2 out]
            n60 = property class="App"() -> ("App.Kind"=w162:T2)  [unwired: 2 in, 2 out]
            n61 = Not(x=w163) -> (.not. x?=w160:bool)
            n62 = Equal?(x=w162, y=T2."Run Time System" ("Application:Kind")) -> (x = y?=w159:bool)
            n63 = Or(x=w160, y=w159) -> ()  [unwired: 1 out]
          }
          frame Enabled {
          }
        }
        n64 = control-ref of="Current VI Reference"() -> (w153:refnum<vi>)
        n65 = Bundle By Name(cluster=w154, "Core.Current VI Reference"=w153, "Core.Close Panel on Exit?"=FALSE) -> (w156:T6)
        n66 = call <vilib>:"Add State(s) to Queue__JKI_lib_State_Machine.vi"("State(s) in (\"\")"=w158) -> ("States Out"=w157:string)  [unwired: 14 in]
      }
      frame "Error Handler" {
        # "Handle any errors here.\nYou can also output any states to clean-up after errors occur"
        n67 = Unbundle By Name(w167) -> ("source"=w166:string)
        n68 = Format Into String(format string="UI: Update Status >> %s\nUI: Cursor Set >> Idle\nClose Equipment Resources", error in=w167, w166) -> (resulting string=w164:string, error out=w169:errorcluster)  [unwired: 1 in]
        n69 = call <vilib>:"Clear Errors.vi"("error in (no error)"=w169) -> ("error out"=w168:errorcluster)  [unwired: 5 in, 1 out]
        n70 = call <vilib>:"Add State(s) to Queue__JKI_lib_State_Machine.vi"("State(s) in Front (\"\")"=w164, "State(s) in (\"\")"=w173) -> ("States Out"=w172:string)  [unwired: 13 in]
      }
      frame "Exit" {
      }
      frame "Stop" {
        w180 = TRUE
        n71 = Stop(stop? (T)=w180) -> ()
      }
      frame "---------- Data ----------" {
        # "Do not put any code in this frame.\n(It is a separator no-op. You can make a copy of this frame to create a new Data frame)"
        n72 = call <vilib>:"Add State(s) to Queue__JKI_lib_State_Machine.vi"("State(s) in (\"\")"=w188) -> ("States Out"=w187:string)  [unwired: 14 in]
      }
      frame "Data: Initialize" {
        w190 = T7 {"Current VI Reference"=refnum, "Close Panel on Exit?"=FALSE}  # Core
        w192 = TRUE  # Your Boolean data
        w191 = ""  # Your string data
        # "do not delete - used by framework"
        # "Expand Bundle to add new data elements to shift register data."
        # "Add new data here."
        # "Data names and types of shift register data are defined by this bundle."
        # "Initialize the shift-register data, here.\n(data names are defined by what you wire into the bundle function)"
        n73 = Bundle("Core"=w190, "Your Boolean data"=w192, "Your string data"=w191) -> (w194:T6)  [unwired: 1 in]
        n74 = call <vilib>:"Add State(s) to Queue__JKI_lib_State_Machine.vi"("State(s) in (\"\")"=w196) -> ("States Out"=w195:string)  [unwired: 14 in]
      }
      frame "Data: Cleanup" {
        # "Cleanup any data and references, here.\n(this is called automatically, by the Macro: Exit)"
        n75 = Unbundle By Name(w198) -> ("Core.Current VI Reference"=w201:refnum<vi>)
        n76 = Close Reference(reference=w201, error in (no error)=w200) -> (error out=w199:errorcluster)
        n77 = call <vilib>:"Add State(s) to Queue__JKI_lib_State_Machine.vi"("State(s) in (\"\")"=w203) -> ("States Out"=w202:string)  [unwired: 14 in]
      }
      frame "---------- UI ----------" {
        # "Do not put any code in this frame.\n(It is a separator no-op. You can make a copy of this frame to create a new UI frame)"
        n78 = call <vilib>:"Add State(s) to Queue__JKI_lib_State_Machine.vi"("State(s) in (\"\")"=w208) -> ("States Out"=w207:string)  [unwired: 14 in]
      }
      frame "UI: Initialize" {
        # "Initialize the User Interface, here.\n(this is called automatically, by the Macro: Init)"
        n79 = call <vilib>:"Add State(s) to Queue__JKI_lib_State_Machine.vi"("State(s) in (\"\")"=w213) -> ("States Out"=w212:string)  [unwired: 14 in]
      }
      frame "UI: Cursor Set" {
        # "Argument"
        # "Set and Unset Cursor Busy.\n(Usage: \"UI: Cursor Set >> Busy|Idle\")"
        n80 = case shown="\"Idle\", Default" w215 {
          tunnel: w217 -> [w222 w224]
          tunnel: [w221 w223] -> w216
          frame "Idle", Default {
            n81 = call <vilib>:"Unset Busy.vi"("error in (no error)"=w222) -> ("error out"=w221:errorcluster)  [unwired: 10 in]
          }
          frame "Busy" {
            n82 = call <vilib>:"Set Busy.vi"("error in (no error)"=w224) -> ("error out"=w223:errorcluster)  [unwired: 9 in, 1 out]
          }
        }
        n83 = call <vilib>:"Add State(s) to Queue__JKI_lib_State_Machine.vi"("State(s) in (\"\")"=w220) -> ("States Out"=w219:string)  [unwired: 14 in]
      }
      frame "UI: Front Panel State" {
        # "Argument"
        # "Set Front Panel Open or Closed\n(Usage: \"UI: Front Panel State >> Open|Close\")"
        n84 = Unbundle By Name(w228) -> ("Core.Current VI Reference"=w227:refnum<vi>)
        n85 = case shown="\"Open\", Default" w226 {
          tunnel: w230 -> [w236 w249]
          tunnel: [w238 w250] -> w229
          tunnel: w227 -> [w237 w247]
          frame "Open", Default {
            n86 = property class="VI"(reference=w237, error in=w236) -> (reference out=w234:refnum<vi>, error out=w235:errorcluster, "Front Panel.Open"=w233:bool)
            n87 = case shown="True" w233 {
              tunnel: [w241 w244] -> w238
              tunnel: w235 -> [w240 w244]
              tunnel: w234 -> [w239 _]
              frame False {
                n88 = invoke class="VI" method="FP.Open"(reference=w239, error in=w240, "Activate"=TRUE, "State"=T3."Standard") -> (error out=w241:errorcluster)  [unwired: 1 in, 4 out]
              }
              frame True {
              }
            }
          }
          frame "Close" {
            n89 = property class="VI"(reference=w247, error in=w249) -> (reference out=w246:refnum<vi>, error out=w248:errorcluster, "Front Panel.Open"=w245:bool)
            n90 = case shown="True" w245 {
              tunnel: [w251 w254] -> w250
              tunnel: w248 -> [w251 w253]
              tunnel: w246 -> [_ w252]
              frame False {
              }
              frame True {
                n91 = invoke class="VI" method="FP.Close"(reference=w252, error in=w253) -> (error out=w254:errorcluster)  [unwired: 1 in, 2 out]
              }
            }
          }
        }
        n92 = call <vilib>:"Add State(s) to Queue__JKI_lib_State_Machine.vi"("State(s) in (\"\")"=w232) -> ("States Out"=w231:string)  [unwired: 14 in]
      }
      frame "UI: Update Status" {
        n93 = local write "Status"(w256) -> ()
      }
      frame "---------- Macro ----------" {
        # "Do not put any code in this frame.\n(It is a separator no-op. You can make a copy of this frame to create a new Macro frame)"
        n94 = call <vilib>:"Add State(s) to Queue__JKI_lib_State_Machine.vi"("State(s) in (\"\")"=w264) -> ("States Out"=w263:string)  [unwired: 14 in]
      }
      frame "Macro: Initialize" {
        w286 = path ""  # INI Path
        w303 = 0 items=["dBm", "W"] ("Unit (0: dBm)")
        w289 = T8 {"Channel (1)"=1, "Avg Count"=10, "Correction Frequency"=10000000.0, "Timeout"=1000, "Reset Device"=FALSE, "ID Query"=FALSE, "Resource Name"="PM1", "Ref Level (dB)"=0.0}  # Input parameters
        w293 = 0.0 ("Frequency (Hz)")
        w297 = 1  # Avg Count
        w318 = "Data: Initialize\nInitialize Core Data\nUI: Initialize\nUI: Front Panel State >> Open\nRead Config INI\nUI: Update Status >> Press [Start] button to start cal. Press [Abort] button to cancel. Update Configuration INI here.\nUI: Cursor Set >> Idle"  # Data: Initialize Initialize Core Data UI: Initialize UI: Front Panel State >> Open Read Config INI UI: Update Status >> Press [Start] button to start cal. Press [Abort] button to cancel. Update Configuration INI here. UI: Cursor Set >> Idle
        w299 = cluster{dbl[]}[] [{[]}, {[]}, {[]}, {[]}]  # Path Loss
        w309 = ""  # Status
        w310 = dbl[] []  # Input Path Loss
        w311 = dbl[] []  # Cal Freqs
        w312 = 10000000.0  # Initial Cal Freq
        w313 = 0  # Rows
        # "// This is the initial state called when VI is run.\n// Initialize main variables and master cluster used for passing values between states/pages."
        n95 = case shown="False" "Secure Display" {
          tunnel: w291 -> [w325 w329]
          tunnel: [w324 w328] -> w290
          frame True {
            w322 = T9."Disabled and Grayed Out" ("Disabled")
            n96 = property on="Frequency (Hz)" class="DigNum (strict)"(error in=w325, "DisabledEnum"=w322) -> (error out=w323:errorcluster)  [unwired: 1 in, 1 out]
            n97 = property on="Corrected Pwr (dBm)" class="DigNum (strict)"(error in=w323, "DisabledEnum"=w322) -> (error out=w324:errorcluster)  [unwired: 1 in, 1 out]
          }
          frame False {
            w326 = T9."Enabled" ("Disabled")
            n98 = property on="Frequency (Hz)" class="DigNum (strict)"(error in=w329, "DisabledEnum"=w326) -> (error out=w327:errorcluster)  [unwired: 1 in, 1 out]
            n99 = property on="Corrected Pwr (dBm)" class="DigNum (strict)"(error in=w327, "DisabledEnum"=w326) -> (error out=w328:errorcluster)  [unwired: 1 in, 1 out]
          }
        }
        n100 = property on="Start" class="Bool (strict)"(error in=w290, "Visible"=TRUE) -> (error out=w298:errorcluster)  [unwired: 1 in, 1 out]
        n101 = property on="Stop" class="Bool (strict)"(error in=w298, "Visible"=FALSE) -> (error out=w277:errorcluster)  [unwired: 1 in, 1 out]
        n102 = Bundle(cluster=w316, "INI Path"=w286, "PSA E4440A GPIB"="PSA E4440A GPIB", "EPM GPIB ALIAS"="EPM GPIB ALIAS", "U2000 GPIB ALIAS"="U2000 GPIB ALIAS", "SigGen (ESG)"="SigGen (ESG)", "SigGen (RFSG)"="SigGen (RFSG)", "Power Level Ref-ESG(dBm)"="Power Level Ref-ESG(dBm)", "Power Level - RFSG(dBm)"="Power Level - RFSG(dBm)", "Initial Cal Freq"=w312, "Span (Hz)"="Span (Hz)", "Cal Freqs"=w311, "Input Path Loss"=w310, "ALC"="ALC", "PM State"="PM State", "Freq Mode"="Freq Mode", "Zero Span"="Zero Span", "SG_Type"="SG_Type", "PM Type"="PM Type", "Channel"="Channel", "Avg Count"=w297, "Measurement Speed"="Measurement Speed", "Measuring Function"="Measuring Function", "Sensor 1 Channel"="Sensor 1 Channel", "Sensor 2 Channel"="Sensor 2 Channel", "Unit (0: dBm)"=w303, "Rows"=w313, "Normalization Files"=path[] [path "\\\\raven\\groups/Programs/TACMAN/Software/AldrinA_Test_Apps/AMCTRDVRFCCA/Calibration/SG2-zero.csv"], "Path Loss"=w299, "Input parameters"=w289, "Status"=w309) -> (w275:T5)
        n103 = control-ref of="This VI"() -> (w276:refnum<vi>)
        n104 = property class="VI"(reference=w276, error in=w277) -> (error out=w283:errorcluster, "Name"=w282:string)  [unwired: 1 out]
        n105 = Match Pattern(string=w282, regular expression="[.]" ("search string")) -> (before substring=w281:string)  [unwired: 1 in, 3 out]
        n106 = Format Into String(format string="%s_Config.ini", error in=w283, w281) -> (resulting string=w279:string, error out=w272:errorcluster)  [unwired: 1 in]
        n107 = call "Utility Create Data Directory.vi"("Folder Name"="Config Files") -> ("Path"=w285:path)  [unwired: 2 in]
        n108 = Build Path(base path=w285, name or relative path=w279) -> (appended path=w273:path)
        n109 = Bundle By Name(cluster=w275, "INI Path"=w273) -> (w274:T5)
        n110 = call <vilib>:"Add State(s) to Queue__JKI_lib_State_Machine.vi"("State(s) in Front (\"\")"=w318, "State(s) in (\"\")"=w321) -> ("States Out"=w320:string)  [unwired: 13 in]
        "Status" <- ""
        "Frequency (Hz)" <- w293
        "Corrected Pwr (dBm)" <- w293
      }
      frame "Macro: Exit" {
        # "Exit Macro\n(This is called once, when the VI exits)"
        n111 = Unbundle By Name(w337) -> ("Core.Close Panel on Exit?"=w336:bool)
        n112 = Select(t="UI: Front Panel State >> Close", s=w336, f="") -> (s? t:f=w333:string)
        n113 = call <vilib>:"Add State(s) to Queue__JKI_lib_State_Machine.vi"("State(s) in (\"\")"=w333, "State(s) at Back (\"\")"="Data: Cleanup\nStop") -> ("States Out"=w331:string)  [unwired: 13 in]
        n114 = call <vilib>:"Add State(s) to Queue__JKI_lib_State_Machine.vi"("State(s) in Front (\"\")"=w331, "State(s) in (\"\")"=w340) -> ("States Out"=w339:string)  [unwired: 13 in]
      }
      frame "Init: RFSG" {
        # "Do not put any code in this frame.\n(It is a separator no-op. You can make a copy of this frame to create a new Macro frame)"
        n115 = Unbundle By Name(w352) -> ("Initial Cal Freq"=w348:dbl, "Power Level - RFSG(dBm)"=w349:dbl, "SigGen (RFSG)"=w350:refnum<k15>)
        n116 = case shown="No Error" w351 {
          selector: w351 -> [w392 w400]
          tunnel: [w366 w400] -> w347
          tunnel: w350 -> [w385 w399]
          tunnel: w349 -> [w382 _]
          tunnel: w348 -> [w381 _]
          tunnel: [w365 w399] -> w341
          frame No Error {
            w375 = TRUE
            w384 = 1000 items=["CW"=1000, "Arb Waveform"=1001, "Script"=1002] ("generation mode")
            # "Perform Self-Cal for only the\nRFSG models listed!!"
            n117 = call <instrlib>:"niRFSG Initialize.vi"("resource name"=w385, "id query"=w375, "reset device"=w375, "error in"=w392) -> ("instrument handle"=w374:refnum<k15>, "error out"=w372:errorcluster)  [unwired: 10 in]
            n118 = property class="niRFSG"(reference=w374, error in=w372) -> (reference out=w373:refnum<k15>, error out=w370:errorcluster, "Model"=w371:string)
            n119 = Match First String(2:string[] ["5610", "5670", "5671", "5672", "5673", "5673E", "5840"], 3:w371) -> (0:w368:i32)  [unwired: 1 out]
            n120 = case shown="0..4" w368 {
              tunnel: [w393 w398] -> w380
              tunnel: [w394 w397] -> w379
              tunnel: w373 -> [w393 w396]
              tunnel: w370 -> [w394 w395]
              frame -1, Default {
              }
              frame 0..4 {
                # "Self-Cal only works\nfor certain RFSG\nmodels!!"
                n121 = call <instrlib>:"niRFSG Self Cal.vi"("instrument handle"=w396, "error in"=w395) -> ("instrument handle out"=w398:refnum<k15>, "error out"=w397:errorcluster)  [unwired: 12 in]
              }
            }
            n122 = call <instrlib>:"niRFSG Configure RF.vi"("instrument handle"=w380, "frequency (Hz)"=w381, "power level (dBm)"=w382, "error in"=w379) -> ("instrument handle out"=w388:refnum<k15>, "error out"=w391:errorcluster)  [unwired: 10 in]
            n123 = call <instrlib>:"niRFSG Configure Generation Mode.vi"("instrument handle"=w388, "generation mode"=w384, "error in"=w391) -> ("instrument handle out"=w387:refnum<k15>, "error out"=w390:errorcluster)  [unwired: 11 in]
            n124 = call <instrlib>:"niRFSG Configure Ref Clock.vi"("instrument handle"=w387, "ref clock source"=T4 "PXI_CLK", "ref clock rate (Hz)"=10000000.0, "error in"=w390) -> ("instrument handle out"=w386:refnum<k15>, "error out"=w389:errorcluster)  [unwired: 10 in]
            n125 = call <instrlib>:"niRFSG Initiate.vi"("instrument handle"=w386, "error in"=w389) -> ("instrument handle out"=w377:refnum<k15>, "error out"=w378:errorcluster)  [unwired: 12 in]
            n126 = call <instrlib>:"niRFSG Configure Output Enabled.vi"("instrument handle"=w377, "output enabled"=TRUE, "error in"=w378) -> ("instrument handle out"=w365:refnum<k15>, "error out"=w366:errorcluster)  [unwired: 11 in]
          }
          frame Error {
          }
        }
        n127 = Bundle By Name(cluster=w352, "SigGen (RFSG)"=w341) -> (w342:T5)
        n128 = case shown="No Error" w347 {
          selector: w347 -> [w357 w364]
          tunnel: [w356 w362] -> w346
          tunnel: [w355 w361] -> w343
          tunnel: w345 -> [w358 w360]
          frame No Error {
            n129 = Format Into String(format string="UI: Update Status >> %s Completed", error in=w357, w358) -> (resulting string=w355:string, error out=w356:errorcluster)  [unwired: 1 in]
          }
          frame Error {
            n130 = Format Into String(format string="UI: Update Status >> %s Failed!\nUI: Cursor Set >> Idle\nClose Equipment Resources", error in=w364, w360) -> (resulting string=w361:string, error out=w362:errorcluster)  [unwired: 1 in]
          }
        }
        n131 = call <vilib>:"Add State(s) to Queue__JKI_lib_State_Machine.vi"("State(s) in Front (\"\")"=w343, "State(s) in (\"\")"=w344) -> ("States Out"=w354:string)  [unwired: 13 in]
      }
      frame "Init: SigGen" {
        # "// Initialize Signal Generator 1"
        n132 = Unbundle By Name(w413) -> ("Power Level Ref-ESG(dBm)"=w406:dbl, "SigGen (ESG)"=w412:refnum<visa-resource-name>, "Unit (0: dBm)"=w409:i32, "Freq Mode"=w408:bool)  [unwired: 1 out]
        n133 = call "E443X_ESG_VSG_Initialize.vi"("VISA Resource Name"=w412, "ID Query? (T: Yes)"=FALSE, "Reset? (T: Yes)"=TRUE, "error in (no error)"=w414) -> ("VISA Resource Name Out"=w407:refnum<visa-resource-name>, "error out"=w405:errorcluster)  [unwired: 10 in]
        n134 = case shown="No Error" w405 {
          selector: w405 -> [w429 w452]
          tunnel: w409 -> [w440 _]
          tunnel: w408 -> [w439 _]
          tunnel: w407 -> [w437 _]
          tunnel: [w434 w452] -> w404
          tunnel: w406 -> [w430 _]
          frame No Error {
            w433 = FALSE ("Freq Ref (T:ON)")
            w442 = u16 0 items=["Fixed", "Modulated"] ("Search Reference")
            # "Disable Modulation"
            # "ALC is required"
            # "Ext. Ref CLK is optional since we are using a PM to\nmeasure the Tx carrier."
            n135 = call "E443X_ESG_VSG_OPC.vi"("error in (no error)"=w429, "Wait (1000ms)"=u32 1000, "VISA resource name"=w437) -> ("error out"=w438:errorcluster, "VISA resource name out"=w436:refnum<visa-resource-name>)  [unwired: 7 in]
            n136 = call "E443X_ESG_VSG_Configure_Frequency.vi"("VISA Resource Name"=w436, "Frequency (1000.0)"=50.0 ("Frequency (5E+7 Hz)"), "Freq Ref (T:ON)"=w433, "error in (no error)"=w438, "Freq Mode (T:CW)"=w439) -> ("VISA Resource Name Out"=w445:refnum<visa-resource-name>, "error out"=w444:errorcluster)  [unwired: 9 in]
            n137 = call "E443X_ESG_VSG_Configure_Amplitude.vi"("VISA Resource Name"=w445, "Ampl Ref (F:OFF)"=w433, "Amplitude (-135.00)"=w430, "Unit (0:dBm)"=w440, "Atten Hold (F:OFF)"=w433, "error in (no error)"=w444) -> ("VISA Resource Name Out"=w449:refnum<visa-resource-name>, "error out"=w446:errorcluster)  [unwired: 8 in]
            n138 = call "E443X_ESG_VSG_Enable_Modulation.vi"("VISA Resource Name"=w449, "Status (T:ON)"=w433, "error in (no error)"=w446) -> ("VISA Resource Name Out"=w450:refnum<visa-resource-name>, "error out"=w447:errorcluster)  [unwired: 11 in]
            n139 = call "E443X_ESG_VSG_ALC_Power_Search.vi"("VISA Resource Name"=w450, "ALC BW (T:NORMAL)"="ALC BW", "ALC (T:ON)"=TRUE ("Enable RF Output (F:Disable)"), "Search Reference (0: Fixed)"=w442, "Power Search (F:MANUAL)"="Pwr Srch", "error in (no error)"=w447) -> ("VISA Resource Name Out"=w451:refnum<visa-resource-name>, "error out"=w448:errorcluster)  [unwired: 8 in]
            n140 = call "E443X_ESG_VSG_Enable_RF_Output.vi"("VISA Resource Name"=w451, "Status (T:ON)"=FALSE, "error in (no error)"=w448) -> ("error out"=w434:errorcluster)  [unwired: 11 in, 1 out]
          }
          frame Error {
          }
        }
        n141 = case shown="No Error" w404 {
          selector: w404 -> [w420 w427]
          tunnel: [w419 w425] -> w401
          tunnel: [w418 w424] -> w402
          tunnel: w403 -> [w421 w423]
          frame No Error {
            n142 = Format Into String(format string="UI: Update Status >> %s Completed", error in=w420, w421) -> (resulting string=w418:string, error out=w419:errorcluster)  [unwired: 1 in]
          }
          frame Error {
            n143 = Format Into String(format string="UI: Update Status >> %s Failed!\nUI: Cursor Set >> Idle\nClose Equipment Resources", error in=w427, w423) -> (resulting string=w424:string, error out=w425:errorcluster)  [unwired: 1 in]
          }
        }
        n144 = call <vilib>:"Add State(s) to Queue__JKI_lib_State_Machine.vi"("State(s) in Front (\"\")"=w402, "State(s) in (\"\")"=w417) -> ("States Out"=w416:string)  [unwired: 13 in]
      }
      frame "Init: SpecAn" {
        n145 = Unbundle By Name(w467) -> ("PSA E4440A GPIB"=w466:refnum<visa-resource-name>)
        n146 = call "E4440A_PSA_Initialize.vi"("error in (no error)"=w465, "Reset (True)"=TRUE, "ID Query (True)"=FALSE, "VISA resource name"=w466) -> ("error out"=w461:errorcluster, "VISA resource name out"=w460:refnum<visa-resource-name>)  [unwired: 6 in]
        n147 = case shown="True" "Auto Align" {
          tunnel: w461 -> [w483 w494]
          tunnel: w460 -> [w481 w493]
          tunnel: [w482 w485] -> w457
          frame False {
            n148 = call "E4440A_PSA_OPC.vi"("error in (no error)"=w483, "VISA resource name"=w481) -> ("error out"=w482:errorcluster)  [unwired: 8 in, 1 out]
          }
          frame True {
            # "// waits cal to complete\n// takes ~37s"
            # "// perform self-cal each time we start test"
            n149 = call "Send SCPI command.vi"("Send SCPI Command"="*CAL?;", "error in (no error)"=w494, "VISA resource name"=w493) -> ("error out"=w490:errorcluster, "VISA resource name out"=w484:refnum<visa-resource-name>)  [unwired: 7 in]
            n150 = property on="Status" class="Str"(error in=w490, "Value"="Calibrating Spectrum Analyzer.\nPlease Wait.", "Blinking"=TRUE) -> (error out=w489:errorcluster)  [unwired: 1 in, 1 out]
            n151 = call "Utility Wait.vi"("Error In"=w489, "Wait (ms)"=u32 38000) -> ("Error Out"=w486:errorcluster)  [unwired: 17 in]
            n152 = call "E4440A_PSA_OPC.vi"("error in (no error)"=w486, "VISA resource name"=w484) -> ("error out"=w485:errorcluster)  [unwired: 8 in, 1 out]
          }
        }
        n153 = case shown="Error" w457 {
          selector: w457 -> [w473 w480]
          tunnel: [w472 w478] -> w454
          tunnel: [w471 w477] -> w455
          tunnel: w456 -> [w474 w476]
          frame No Error {
            n154 = Format Into String(format string="UI: Update Status >> %s Completed", error in=w473, w474) -> (resulting string=w471:string, error out=w472:errorcluster)  [unwired: 1 in]
          }
          frame Error {
            n155 = Format Into String(format string="UI: Update Status >> %s Failed!\nUI: Cursor Set >> Idle\nClose Equipment Resources", error in=w480, w476) -> (resulting string=w477:string, error out=w478:errorcluster)  [unwired: 1 in]
          }
        }
        n156 = property on="Status" class="Str"(error in=w454, "Value"="Spectrum Analyzer Self-Calibration Done." ("Status"), "Blinking"=FALSE) -> (error out=w453:errorcluster)  [unwired: 1 in, 1 out]
        n157 = call <vilib>:"Add State(s) to Queue__JKI_lib_State_Machine.vi"("State(s) in Front (\"\")"=w455, "State(s) in (\"\")"=w459) -> ("States Out"=w458:string)  [unwired: 13 in]
      }
      frame "Config: SpecAn" {
        w507 = u16 0 items=["dBm", "dBmV", "dBmA", "dBuV", "dBuVm", "dBuA", "dBuAm", "dBpt", "dBg", "Volts", "Watts", "Amps"] ("Amplitude Units (0: dBm)")
        w513 = u16 0 items=["Auto", "RMS", "Video", "Scalar"] ("Averaging Type (0: Auto)")
        n158 = Unbundle By Name(w502) -> ("PSA E4440A GPIB"=w529:refnum<visa-resource-name>, "Initial Cal Freq"=w506:dbl, "Span (Hz)"=w505:dbl)
        n159 = call "Send SCPI command.vi"("Send SCPI Command"=":DET:NORM;\n:TRAC1:MODE WRIT;\n:INP:COUP AC;\n:FREQ:OFFS 0.00;\n:CALC:MARK:AOFF;\n:CALC:MARK:TABL:STAT OFF;\n:TRIG:SLOP POS;", "error in (no error)"=w528, "VISA resource name"=w529) -> ("error out"=w527:errorcluster, "VISA resource name out"=w523:refnum<visa-resource-name>)  [unwired: 7 in]
        n160 = case shown="\"Auto\"" "SpecAn Mode" {
          tunnel: ["VBW (Hz)" _] -> w511
          tunnel: ["RBW (Hz)" _] -> w510
          tunnel: [FALSE ("Enable Auto Video BandWidth (T: Enable)") TRUE ("Enable Auto Video BandWidth (T: Enable)")] -> w509
          frame "Manual", Default {
          }
          frame "Auto" {
          }
        }
        n161 = call "E4440A_PSA_Center_Span.vi"("error in (no error)"=w527, "Span (2 GHz)"=w505, "Center Frequency (2 GHz)"=w506, "VISA resource name"=w523) -> ("error out"=w522:errorcluster, "VISA resource name out"=w521:refnum<visa-resource-name>)  [unwired: 6 in]
        n162 = call "E4440A_PSA_Sweep_Coupling.vi"("VISA resource name"=w521, "Enable Auto Video BandWidth (T: Enable)"=w509, "Manual Video BandWidth (3 MHz)"=w511, "Enable Auto Sweep Time (T: Enable)"=w509, "Enable Auto Resolution BandWidth (T: Enable)"=w509, "error in (no error)"=w522, "Manual Resolution BandWidth (3 MHz)"=w510, "Enable Auto VBW/RBW Ratio (T: Enable)"=w509) -> ("VISA resource name out"=w519:refnum<visa-resource-name>, "error out"=w520:errorcluster)  [unwired: 6 in]
        n163 = call "E4440A_PSA_Configure_Level.vi"("VISA resource name"=w519, "Reference Level (0)"="Ref Lvl (dBm)", "Amplitude Units (0: dBm)"=w507, "error in (no error)"=w520, "Enable Auto Attenuation (T: Enable)"="Auto Atten", "Manual Attenuation (30 dB)"="Atten (dB)", "Attenuation Step (2 dB)"=2 ("Step (dB)")) -> ("VISA resource name out"=w503:refnum<visa-resource-name>, "error out"=w504:errorcluster)  [unwired: 7 in]
        n164 = Unbundle By Name(w502) -> ("Zero Span"=w501:bool)
        n165 = call "E4440A_PSA_Averaging.vi"("Enable Averaging (T: Enable)"="Averaging", "error in (no error)"=w504, "Averaging Type (0: Auto)"=w513, "Average Count (100)"="Avg", "VISA resource name"=w503) -> ("error out"=w526:errorcluster, "VISA resource name out"=w524:refnum<visa-resource-name>)  [unwired: 5 in]
        n166 = case shown="False" w501 {
          tunnel: w526 -> [w544 w548]
          tunnel: [w542 w546] -> w500
          tunnel: w524 -> [w541 w545]
          frame False {
            n167 = call "Send SCPI command.vi"("Send SCPI Command"=":INIT:CONT ON;\n:INIT:IMM;" ("multi-line string"), "error in (no error)"=w544, "VISA resource name"=w541) -> ("error out"=w542:errorcluster)  [unwired: 7 in, 1 out]
          }
          frame True {
            n168 = call "Send SCPI command.vi"("Send SCPI Command"=":FREQ:SPAN 0 Hz;\n:INIT:CONT ON;\n:INIT:IMM;" ("multi-line string"), "error in (no error)"=w548, "VISA resource name"=w545) -> ("error out"=w546:errorcluster)  [unwired: 7 in, 1 out]
          }
        }
        n169 = case shown="Error" w500 {
          selector: w500 -> [w533 w540]
          tunnel: [w532 w538] -> w499
          tunnel: [w531 w537] -> w495
          tunnel: w498 -> [w534 w536]
          frame No Error {
            n170 = Format Into String(format string="UI: Update Status >> %s Completed", error in=w533, w534) -> (resulting string=w531:string, error out=w532:errorcluster)  [unwired: 1 in]
          }
          frame Error {
            n171 = Format Into String(format string="UI: Update Status >> %s Failed!\nUI: Cursor Set >> Idle\nClose Equipment Resources", error in=w540, w536) -> (resulting string=w537:string, error out=w538:errorcluster)  [unwired: 1 in]
          }
        }
        n172 = call <vilib>:"Add State(s) to Queue__JKI_lib_State_Machine.vi"("State(s) in Front (\"\")"=w495, "State(s) in (\"\")"=w497) -> ("States Out"=w496:string)  [unwired: 13 in]
      }
      frame "Init: E44xx Power Meter" {
        # "// Initialize Power Meter"
        n173 = call <vilib>:"Three Button Dialog.vi"("Window Title (\"\")"="Power Meter Calibration" ("Window Title (\"\")"), "message"="Zero + Cal Power Head\nCompleted?") -> ("Which Button?"=w555:T10)  [unwired: 9 in]
        n174 = Unbundle By Name(w581) -> ("Channel"=w577:i32, "PM State"=w571:bool, "Avg Count"=w568:i32, "Sensor 1 Channel"=w570:i32, "Sensor 2 Channel"=w569:i32, "Measuring Function"=w572:i32, "EPM GPIB ALIAS"=w580:refnum<visa-resource-name>, "Unit (0: dBm)"=w567:i32)
        n175 = case shown="\"Center Button\", Default" w555 {
          tunnel: w554 -> [w587 w591]
          tunnel: [w587 w592] -> w553
          frame "Left Button" {
            # "YES"
          }
          frame "Center Button", Default {
            # "NO"
            n176 = Bundle By Name(cluster=w591, "status"=TRUE, "code"=1, "source"="Zero + Cal Required") -> (w592:errorcluster)
          }
        }
        n177 = call "E441X_PM_Initialize.vi"("Instrument Resource Name"=w580, "ID Query (T: Check)"=FALSE, "Reset (T: Reset)"=TRUE, "error in (no error)"=w553) -> ("VISA session"=w582:refnum<visa-resource-name>, "error out"=w560:errorcluster)  [unwired: 10 in]
        n178 = call "Utility Wait.vi"("Error In"=w560, "Wait (ms)"=u32 5000) -> ("Error Out"=w559:errorcluster)  [unwired: 17 in]
        n179 = Index Array(array=i32[] [1, 2], index=w577) -> (element=w573:i32)
        n180 = case shown="No Error" w559 {
          selector: w559 -> [w594 w617]
          tunnel: w582 -> [w606 _]
          tunnel: [w605 w617] -> w575
          tunnel: w573 -> [w600 _]
          tunnel: w572 -> [w599 _]
          tunnel: w571 -> [w593 _]
          tunnel: w570 -> [w598 _]
          tunnel: w569 -> [w597 _]
          tunnel: w568 -> [w596 _]
          tunnel: w567 -> [w595 _]
          frame No Error {
            w616 = 0 items=["Single", "Single Relative", "Difference", "Difference Relative", "Ratio", "Ratio Relative"] ("Measuring Function (0: Single)")
            w613 = 0 items=["Immediate", "Bus", "Hold", "External", "Internal A", "Internal B"] ("Source (0: Immediate)")
            n181 = call "E441X_PM_Configure_Measurement.vi"("VISA session"=w606, "Measurement (1)"=w600, "Measuring Function (0: Single)"=w599, "Sensor 1 (0: Channel A)"=w598, "Sensor 2 (0: Channel A)"=w597, "error in (no error)"=w594, "Resolution (3)"="Resolution", "Unit (0: dBm)"=w595) -> ("dup VISA session"=w610:refnum<visa-resource-name>, "error out"=w608:errorcluster)  [unwired: 6 in]
            n182 = call "E441X_PM_Configure_Limits.vi"("VISA session"=w610, "Measurement (1)"=w600, "State (T: On)"=w593, "Auto Clear (1: On)"="Auto Clear", "error in (no error)"=w608) -> ("dup VISA session"=w603:refnum<visa-resource-name>, "error out"=w604:errorcluster)  [unwired: 9 in]
            n183 = call "E441X_PM_Configure_Averaging.vi"("VISA session"=w603, "Channel (0: A)"=w600, "State (T: On)"=w593, "Filter Length (4)"=w596, "error in (no error)"=w604) -> ("dup VISA session"=w601:refnum<visa-resource-name>, "error out"=w602:errorcluster)  [unwired: 9 in]
            n184 = call "E441X_PM_Set_Initiate_Continuous_State.vi"("VISA session"=w601, "Channel (0: A)"=w600, "State (T: On)"=w593, "error in (no error)"=w602) -> ("dup VISA session"=w611:refnum<visa-resource-name>, "error out"=w609:errorcluster)  [unwired: 10 in]
            n185 = call "E441X_PM_Configure_Trigger.vi"("VISA session"=w611, "Channel (0: A)"=w600, "Delay Auto State (T: On)"=w593, "Source (0: Immediate)"=w613, "error in (no error)"=w609) -> ("dup VISA session"=w615:refnum<visa-resource-name>, "error out"=w614:errorcluster)  [unwired: 9 in]
            n186 = call "E441X_PM_Read_Measurement.vi"("VISA session"=w615, "Measurement (1)"=w600, "Measuring Function (0: Single)"=w616, "error in (no error)"=w614) -> ("error out"=w605:errorcluster)  [unwired: 9 in, 2 out]
          }
          frame Error {
          }
        }
        n187 = Greater?(x="Avg Count", y=1) -> (0:w561:bool)
        n188 = case shown="False" w561 {
          tunnel: [1 ("Averaging Count") w619] -> w564
          tunnel: "Avg Count" -> [_ w619]
          frame False {
          }
          frame True {
          }
        }
        n189 = case shown="Error" w575 {
          selector: w575 -> [w622 w629]
          tunnel: [w621 w627] -> w576
          tunnel: [w620 w626] -> w574
          tunnel: w566 -> [w623 w625]
          frame No Error {
            n190 = Format Into String(format string="UI: Update Status >> %s Completed", error in=w622, w623) -> (resulting string=w620:string, error out=w621:errorcluster)  [unwired: 1 in]
          }
          frame Error {
            n191 = Format Into String(format string="UI: Update Status >> %s Failed!\nUI: Cursor Set >> Idle\nClose Equipment Resources", error in=w629, w625) -> (resulting string=w626:string, error out=w627:errorcluster)  [unwired: 1 in]
          }
        }
        n192 = Bundle By Name(cluster=w581, "Avg Count"=w564) -> (w565:T5)
        n193 = call <vilib>:"Add State(s) to Queue__JKI_lib_State_Machine.vi"("State(s) in Front (\"\")"=w574, "State(s) in (\"\")"=w586) -> ("States Out"=w585:string)  [unwired: 13 in]
      }
      frame "Init: U20000 Power Meter" {
        # "// Initialize Power Meter"
        n194 = Unbundle By Name(w647) -> ("U2000 GPIB ALIAS"=w643:refnum<visa-resource-name>)
        n195 = call "U2000_USB_PM_Initialize.vi"("error in (no error)"=w644, "Reset (True)"=TRUE ("Reset (T: Reset)"), "ID Query (True)"=FALSE ("ID Query (T: Check)"), "VISA resource name"=w643) -> ("error out"=w632:errorcluster, "VISA resource name out"=w634:refnum<visa-resource-name>)  [unwired: 6 in]
        n196 = call "U2000_USB_PM_OPC.vi"("error in (no error)"=w632, "VISA resource name"=w634) -> ("error out"=w631:errorcluster, "VISA resource name out"=w633:refnum<visa-resource-name>)  [unwired: 8 in]
        n197 = case shown="No Error" w631 {
          selector: w631 -> [w659 w675]
          tunnel: w633 -> [w658 w674]
          tunnel: [w660 w675] -> w635
          tunnel: [w651 w674] -> w630
          frame No Error {
            w662 = 1 items=["Calculate Block 1"=1, "Calculate Block 2"=2, "Calculate Block 3"=3, "Calculate Block 4"=4] ("Calculate Block (1: Calculate Block 1)")
            n198 = call "U2000_USB_PM_Configure_Cal_Zero.vi"("Zero Mode"=enum16{"ONCE", "ON", "OFF"}."ON", "Cal Mode"=enum16{"ONCE", "OFF", "ON"}."ON", "error in (no error)"=w659, "Cal ALL [F]"=TRUE, "VISA resource name"=w658) -> ("error out"=w654:errorcluster, "VISA resource name out"=w655:refnum<visa-resource-name>)  [unwired: 4 in, 1 out]
            n199 = call "U2000_USB_PM_Configure_Units.vi"("Calculate Block (1: Calculate Block 1)"=w662, "error in (no error)"=w654, "Units (0: dBm)"="Units", "VISA resource name"=w655) -> ("error out"=w672:errorcluster, "VISA resource name out"=w671:refnum<visa-resource-name>)  [unwired: 6 in]
            n200 = call "U2000_USB_PM_Configure_Trigger.vi"("VISA resource name"=w671, "Trigger Count (1)"=1, "Trigger Level (0 dBm)"="Trigger Level (dBm)", "Trigger Slope (0: Positive)"="Trigger Slope", "Trigger Source (3: Immediate)"="Trigger Source", "error in (no error)"=w672) -> ("VISA resource name out"=w669:refnum<visa-resource-name>, "error out"=w670:errorcluster)  [unwired: 8 in]
            n201 = call "U2000_USB_PM_Enable_Initiate_Continuous.vi"("Enable Initiate Continuous (T: Enable)"=TRUE ("Enable Initiate Continuous"), "error in (no error)"=w670, "VISA resource name"=w669) -> ("error out"=w667:errorcluster, "VISA resource name out"=w668:refnum<visa-resource-name>)  [unwired: 7 in]
            n202 = call "U2000_USB_PM_Configure_Correction.vi"("error in (no error)"=w667, "Frequency (5E+7 Hz)"=50000000.0, "VISA resource name"=w668) -> ("error out"=w660:errorcluster, "VISA resource name out"=w651:refnum<visa-resource-name>)  [unwired: 7 in]
          }
          frame Error {
          }
        }
        n203 = case shown="False" "Enable Averaging" {
          tunnel: [1 ("Averaging Count") w677] -> w636
          tunnel: "Averaging Count" -> [_ w677]
          frame False {
          }
          frame True {
          }
        }
        n204 = case shown="No Error" w635 {
          selector: w635 -> [w680 w687]
          tunnel: [w679 w686] -> w646
          tunnel: [w678 w683] -> w645
          tunnel: w640 -> [w681 w685]
          frame No Error {
            n205 = Format Into String(format string="UI: Update Status >> %s Completed", error in=w680, w681) -> (resulting string=w678:string, error out=w679:errorcluster)  [unwired: 1 in]
          }
          frame Error {
            n206 = Format Into String(format string="UI: Update Status >> %s Failed!\nUI: Cursor Set >> Idle\nClose Equipment Resources", error in=w687, w685) -> (resulting string=w683:string, error out=w686:errorcluster)  [unwired: 1 in]
          }
        }
        n207 = Bundle By Name(cluster=w647, "Avg Count"=w636, "U2000 GPIB ALIAS"=w630) -> (w639:T5)
        n208 = call <vilib>:"Add State(s) to Queue__JKI_lib_State_Machine.vi"("State(s) in Front (\"\")"=w645, "State(s) in (\"\")"=w650) -> ("States Out"=w649:string)  [unwired: 13 in]
      }
      frame "---------- New Category ----------" {
        # "Template Separator\n(You can make a copy of, or modify, this frame)"
        n209 = call <vilib>:"Add State(s) to Queue__jki_lib_state_machine.vi"("State(s) in (\"\")"=w692) -> ("States Out"=w691:string)  [unwired: 14 in]
      }
      frame "Save Config INI" {
        # "// Save control values & states to INI file\n// Config.INI saved in directory as this VI"
        n210 = Unbundle By Name(w698) -> ("INI Path"=w697:path)
        n211 = control-ref of="This VI"() -> (w696:refnum<vi>)
        n212 = call "Utility Write Config INI to File.vi"("File Type"=".ini", "Error In"=w700, "reference"=w696, "Path In"=w697) -> ("Error Out"=w699:errorcluster, "Path Out"=w694:path)  [unwired: 6 in]
        n213 = Path To String(path=w694) -> (string=w693:string)
        n214 = Concatenate Strings("UI: Update Status >> Configuration INI Saved to: " ("State(s) in Front (\"\")"), w693) -> (w701:string)
        n215 = call <vilib>:"Add State(s) to Queue__JKI_lib_State_Machine.vi"("State(s) in Front (\"\")"=w701, "State(s) in (\"\")"=w705) -> ("States Out"=w704:string)  [unwired: 13 in]
      }
      frame "Read Config INI" {
        # "// Read Config.INI and modifies control values & states from INI file\n// Config.INI saved in directory as this VI"
        n216 = Unbundle By Name(w709) -> ("INI Path"=w708:path)
        n217 = control-ref of="This VI"() -> (w710:refnum<vi>)
        n218 = call "Utility Load Config INI from File.vi"("File Type"=".ini", "Error In"=w713, "reference"=w710, "Path In"=w708) -> ("Error Out"=w712:errorcluster, "Path Out"=w707:path)  [unwired: 6 in]
        n219 = Path To String(path=w707) -> (string=w706:string)
        n220 = Concatenate Strings("UI: Update Status >> Configuration INI read from: " ("State(s) in Front (\"\")"), w706) -> (w716:string)
        n221 = property on="Start" class="Bool (strict)"(error in=w712, "Blinking"=TRUE) -> (error out=w715:errorcluster)  [unwired: 1 in, 1 out]
        n222 = call <vilib>:"Add State(s) to Queue__JKI_lib_State_Machine.vi"("State(s) in Front (\"\")"=w716, "State(s) in (\"\")"=w720) -> ("States Out"=w719:string)  [unwired: 13 in]
      }
      frame "Display Cal Diagrams" {
        # "// Help nags"
        n223 = call "Picture Prompt_Typical_Calibration.vi"("error in (no error)"=w723) -> ("error out"=w724:errorcluster)  [unwired: 9 in, 1 out]
        n224 = call "Picture Prompt_IP3_Calibration.vi"("error in (no error)"=w724) -> ("error out"=w722:errorcluster)  [unwired: 9 in, 1 out]
      }
      frame "Load Normalization Files" {
        # "// CALC PATH LOSS sub-VI will actually do the normalization file(s) loading\n// and determine normalized power."
        n225 = case shown="No Error" w731 {
          selector: w731 -> [w736 w744]
          tunnel: [w735 w742] -> w730
          tunnel: [w738 w740] -> w729
          tunnel: w728 -> [w737 w743]
          frame No Error {
            n226 = Format Into String(format string="UI: Update Status >> %s completed\nBuild Cal Freq Table", error in=w736, w737) -> (resulting string=w738:string, error out=w735:errorcluster)  [unwired: 1 in]
          }
          frame Error {
            n227 = Format Into String(format string="UI: Update Status >> %s Failed!\nUI: Cursor Set >> Idle\nClose Equipment Resources", error in=w744, w743) -> (resulting string=w740:string, error out=w742:errorcluster)  [unwired: 1 in]
          }
        }
        n228 = call <vilib>:"Add State(s) to Queue__JKI_lib_State_Machine.vi"("State(s) in Front (\"\")"=w729, "State(s) in (\"\")"=w734) -> ("States Out"=w733:string)  [unwired: 13 in]
      }
      frame "Build Cal Freq Table" {
        # "how many rows?"
        # "column 0 (Freqs)"
        # "initial freq"
        # "// Load from file or build the lookup table from arbitrary Start, Stop & Intervals"
        n229 = case shown="\"Lookup Table\"" "Tab Control" {
          tunnel: [w779 w795] -> w762
          tunnel: w755 -> [w778 w794]
          tunnel: [w778 w794] -> w754
          frame "Arbitrary", Default {
            n230 = while {
              tunnel: "Stop F (Hz)" -> [w789]
              tunnel: "Intervals (Hz)" -> [w792]
              tunnel: "Start F (Hz)" -> [w793]
              shift-right: [w787] -> w779
              shift-left: dbl[][] [] ("array") -> [w788]
              i -> [w786]
              stop <- w790 stop-if-true
              n231 = Multiply(x=w792, y=w786) -> (x*y=w791:dbl)
              n232 = Add(x=w793, y=w791) -> (x+y=w784:dbl)
              n233 = Build Array(w784) -> (w785:dbl[])
              n234 = Greater?(x=w784, y=w789) -> (0:w790:bool)
              n235 = Insert Into Array(array=w788, index (row)=w786, new element=w785) -> (w787:dbl[][])  [unwired: 1 in]
            }
          }
          frame "Lookup Table" {
            w797 = FALSE  # transpose (no:F)
            n236 = call-poly <vilib>:"Read From Spreadsheet File.vi"("transpose (no:F)"=w797, "file path (dialog if empty)"="file path (dialog if empty)") -> ("all rows"=w795:dbl[][])  [unwired: 5 in, 4 out]
          }
        }
        n237 = Array Size(array=w762) -> (size(s)=w761:i32[])
        n238 = Index Array(array=w762, index (row)=0 ("index"), index (col)=0 ("disabled index (col)")) -> (element=w751:dbl)
        n239 = Index Array(array=w762, index (col)=0 ("disabled index (col)")) -> (element=w750:dbl[])  [unwired: 1 in]
        n240 = Index Array(array=w761, index=0) -> (element=w749:i32)
        n241 = To Double Precision Float(number=w749) -> (double precision float=w758:dbl)
        n242 = property on="Path Loss" class="WFGraph (strict)"(error in=w754, "XScale.Maximum"=w758, "XScale.Minimum"=0.0 ("X Scale.Range:Minimum")) -> (error out=w748:errorcluster)  [unwired: 1 in, 1 out]
        n243 = Bundle By Name(cluster=w753, "Initial Cal Freq"=w751, "Cal Freqs"=w750, "Rows"=w749) -> (w752:T5)
        n244 = case shown="No Error" w748 {
          selector: w748 -> [w769 w776]
          tunnel: [w768 w775] -> w747
          tunnel: [w770 w773] -> w746
          tunnel: w745 -> [w771 w774]
          frame No Error {
            n245 = Format Into String(format string="UI: Update Status >> %s completed\nCalibration Loop", error in=w769, w771) -> (resulting string=w770:string, error out=w768:errorcluster)  [unwired: 1 in]
          }
          frame Error {
            n246 = Format Into String(format string="UI: Update Status >> %s Failed!\nUI: Cursor Set >> Idle\nClose Equipment Resources", error in=w776, w774) -> (resulting string=w773:string, error out=w775:errorcluster)  [unwired: 1 in]
          }
        }
        n247 = call <vilib>:"Add State(s) to Queue__JKI_lib_State_Machine.vi"("State(s) in Front (\"\")"=w746, "State(s) in (\"\")"=w767) -> ("States Out"=w766:string)  [unwired: 13 in]
      }
      frame "Calibration Loop" {
        w804 = cluster{dbl[]}[] []
        w812 = dbl[] []
        # "// automatically enables\n SG amplitude reference\n if there are normalization\n files!!"
        # "// Main loop\n// Signal generator amplitude normalization vs. Frequency cable loss to DUT happens here"
        n248 = Unbundle By Name(w832) -> ("Input parameters"=w806:T8, "Measurement Speed"=w817:i32, "Measuring Function"=w816:i32, "PM State"=w815:bool, "Avg Count"=w818:i32, "Channel"=w825:i32, "PM Type"=w814:T1, "SG_Type"=w799:enum32{"ESG/PSG", "RFSG"}, "EPM GPIB ALIAS"=w819:refnum<visa-resource-name>, "U2000 GPIB ALIAS"=w800:refnum<visa-resource-name>, "PSA E4440A GPIB"=w803:refnum<visa-resource-name>, "SigGen (ESG)"=w831:refnum<visa-resource-name>, "SigGen (RFSG)"=w798:refnum<k15>, "Power Level Ref-ESG(dBm)"=w830:dbl, "Cal Freqs"=w829:dbl[], "Normalization Files"=w810:path[], "Rows"=w826:i32, "Freq Mode"=w813:bool, "Zero Span"=w801:bool, "Span (Hz)"=w802:dbl)
        n249 = Empty Array?(array=w810) -> (empty?=w809:bool)
        n250 = Not(x=w809) -> (.not. x?=w808:bool)
        n251 = Bundle By Name(cluster=w806, "Avg Count"=w818, "Resource Name"=w819) -> (w834:T8)
        n252 = while {
          tunnel: w829 -> [w845] mode=indexing
          tunnel: w826 -> [w896]
          tunnel: w834 -> [w889]
          tunnel: w830 -> [w868]
          tunnel: w819 -> [w890]
          tunnel: w831 -> [w849]
          tunnel: w805 -> [w892]
          tunnel: [w887] -> w821
          shift-right: [w879] -> w827
          shift-left: w812 -> [w893]
          tunnel: w825 -> [w891]
          tunnel: w817 -> [w888]
          tunnel: w816 -> [w885]
          tunnel: w815 -> [w884]
          tunnel: w814 -> [w882]
          tunnel: w813 -> [w850]
          shift-right: [w880] -> _
          shift-left: w812 -> [w881]
          shift-right: [w875] -> _
          shift-left: w812 -> [w877]
          shift-right: [w874] -> _
          shift-left: w812 -> [w876]
          tunnel: w810 -> [w860]
          tunnel: w808 -> [w870]
          shift-right: [w873] -> w811
          shift-left: w804 -> [w864]
          tunnel: w804 -> [w862]
          tunnel: w803 -> [w852]
          tunnel: w802 -> [w858]
          tunnel: w801 -> [w857]
          tunnel: w800 -> [w856]
          tunnel: w799 -> [w854]
          tunnel: w798 -> [w848]
          i -> [w878]
          stop <- w894 stop-if-true
          # "// Enable SG amplitude reference\n// if there are normalization\n// files selected by user."
          # "// Path Loss (dB)"
          # "// SG Pwr Corr\n// Error Factor"
          # "// Measured Pwr"
          # "// Adj SG Pwr"
          # "Delay PM 10ms before read to\nprevent race condition."
          n253 = expression code="X/1000000"(w845) -> (w853:dbl)
          n254 = call "Get Path Loss.vi"("Calibration Enabled"=w870, "Frequency"=w845, "Data File Format"="TwoColumnText", "error in (no error)"=w892, "Power Level"=w868, "Normalization Files"=w860) -> ("error out"=w851:errorcluster, "Adjusted Power Level"=w847:dbl, "Correction Factor (dB)"=w855:dbl, "Route Names"=w859:string[])  [unwired: 1 in, 1 out]
          n255 = case shown="\"RFSG\", Default" w854 {
            tunnel: w847 -> [w912 w918]
            tunnel: w855 -> [w911 _]
            tunnel: w853 -> [w910 _]
            tunnel: w851 -> [w909 w920]
            tunnel: w850 -> [w908 _]
            tunnel: w849 -> [w907 _]
            tunnel: w848 -> [_ w921]
            tunnel: [w900 w919] -> w846
            tunnel: w845 -> [_ w916]
            frame "ESG/PSG" {
              n256 = call "E443X_ESG_VSG_Configure_Frequency.vi"("VISA Resource Name"=w907, "Frequency (1000.0)"=w910, "Freq Ref (T:ON)"=FALSE, "error in (no error)"=w909, "Freq Mode (T:CW)"=w908) -> ("VISA Resource Name Out"=w903:refnum<visa-resource-name>, "error out"=w904:errorcluster)  [unwired: 9 in]
              n257 = call "E443X_ESG_VSG_Configure_Amplitude.vi"("VISA Resource Name"=w903, "Ampl Ref Set (0.00)"=w911, "Amplitude (-135.00)"=w912, "error in (no error)"=w904) -> ("VISA Resource Name Out"=w902:refnum<visa-resource-name>, "error out"=w905:errorcluster)  [unwired: 10 in]
              n258 = call "E443X_ESG_VSG_Enable_RF_Output.vi"("VISA Resource Name"=w902, "Status (T:ON)"=TRUE, "error in (no error)"=w905) -> ("error out"=w901:errorcluster)  [unwired: 11 in, 1 out]
              n259 = call "Utility Wait.vi"("Error In"=w901, "Wait (ms)"=u32 100) -> ("Error Out"=w900:errorcluster)  [unwired: 17 in]
            }
            frame "RFSG", Default {
              n260 = call <instrlib>:"niRFSG Configure RF.vi"("instrument handle"=w921, "frequency (Hz)"=w916, "power level (dBm)"=w918, "error in"=w920) -> ("instrument handle out"=w914:refnum<k15>, "error out"=w915:errorcluster)  [unwired: 10 in]
              n261 = call <instrlib>:"niRFSG Wait Until Settled.vi"("instrument handle"=w914, "Max. time (ms)"=100, "error in"=w915) -> ("error out"=w919:errorcluster)  [unwired: 11 in, 1 out]
            }
          }
          n262 = local read "Secure Display"() -> (w863:bool)
          n263 = case shown="False" w863 {
            tunnel: w845 -> [w927 _]
            tunnel: [w927 nan ("Numeric")] -> w867
            tunnel: [w926 ""] -> w861
            frame False {
              n264 = Format Into String(format string="Measuring: %g Hz", w927) -> (resulting string=w926:string)  [unwired: 2 in, 1 out]
            }
            frame True {
            }
          }
          n265 = case shown="False" w863 {
            tunnel: w864 -> [w922 _]
            tunnel: w862 -> [_ w923]
            frame False {
              "Path Loss" <- w922
            }
            frame True {
              n266 = local write "Path Loss"(w923) -> ()
            }
          }
          n267 = local write "Frequency (Hz)"(w867) -> ()
          n268 = local write "Status"(w861) -> ()
          n269 = Bundle By Name(cluster=w889, "Correction Frequency"=w845) -> (w886:T8)
          n270 = case shown="\"U2000 USB [PM2]\", Default" w882 {
            tunnel: w859 -> [w941 w946 _]
            tunnel: w891 -> [w940 _ _]
            tunnel: w890 -> [w939 _ _]
            tunnel: [w938 w944 w950] -> w865
            tunnel: w888 -> [w937 _ _]
            tunnel: [w936 w947 w954] -> w887
            tunnel: w886 -> [w935 w945 _]
            tunnel: w885 -> [w934 _ _]
            tunnel: w884 -> [w933 _ _]
            tunnel: w846 -> [w932 w948 w955]
            tunnel: FALSE ("Pwr Mtr Cal") -> [w931 w943 _]
            tunnel: w852 -> [_ _ w953]
            tunnel: w845 -> [_ _ w952]
            tunnel: w858 -> [_ _ w951]
            tunnel: w857 -> [_ _ w949]
            tunnel: w856 -> [_ w942 _]
            frame "E44xx EPM [PM1]" {
              n271 = call "Read PM Sensor Channel.vi"("VISA session"=w939, "Measuring Function (0: Single)"=w934, "Measurement Speed"=w937, "Channel (0: A)"=w940, "State (T: On)"=w933, "Input parameters"=w935, "error in"=w932, "Pwr Mtr Cal"=w931, "Route Names"=w941) -> ("dBm"=w938:dbl, "error out"=w936:errorcluster)  [unwired: 4 in, 1 out]
            }
            frame "U2000 USB [PM2]", Default {
              n272 = call "U2044XA Measure RF Power.vi"("Route Names"=w946, "Pwr Mtr Cal"=w943, "error in"=w948, "Input parameters"=w945, "VISA session"=w942) -> ("error out"=w947:errorcluster, "dBm"=w944:dbl)  [unwired: 4 in, 1 out]
            }
            frame "PSA-E444x [E4440]" {
              n273 = call "PSA E4440A Set and Read Marker X and Y Values.vi"("VISA resource name"=w953, "Zero Span"=w949, "error in (no error)"=w955, "Span [Hz]"=w951, "Center Frequency (Hz)"=w952) -> ("Y Amplitude (dBm)"=w950:dbl, "error out"=w954:errorcluster)  [unwired: 7 in, 2 out]
            }
          }
          n274 = case shown="False" w863 {
            tunnel: w865 -> [w924 _]
            tunnel: [w924 nan ("Numeric")] -> w866
            frame False {
            }
            frame True {
            }
          }
          n275 = Subtract(x=w865, y=w868) -> (x-y=w869:dbl)
          n276 = Increment(x=w878) -> (x+1=w895:i32)
          n277 = Insert Into Array(array=w893, index=w878, new element=w869) -> (w879:dbl[])
          n278 = Insert Into Array(array=w881, index=w878, new element=w855) -> (w880:dbl[])
          n279 = Insert Into Array(array=w877, index=w878, new element=w865) -> (w875:dbl[])
          n280 = Insert Into Array(array=w876, index=w878, new element=w847) -> (w874:dbl[])
          n281 = Unbundle By Name(w887) -> ("status"=w898:bool)
          n282 = local read "Stop"() -> (w871:bool)
          n283 = local write "Corrected Pwr (dBm)"(w866) -> ()
          n284 = Greater Or Equal?(x=w895, y=w896) -> (x >= y?=w897:bool)
          n285 = Build Cluster Array(w879, w880, w875, w874) -> (w873:cluster{dbl[]}[])
          n286 = Compound Arithmetic op=OR(w898, w871, w897) -> (w894:bool)
          "Normalization Active" <- w870
        }
        n287 = case shown="No Error" w821 {
          selector: w821 -> [w836 w844]
          tunnel: [w835 w843] -> w820
          tunnel: [w837 w841] -> w822
          tunnel: w807 -> [w838 w840]
          frame No Error {
            n288 = Format Into String(format string="UI: Update Status >> %s completed\nUI: Cursor Set >> Idle\nSave Calibration", error in=w836, w838) -> (resulting string=w837:string, error out=w835:errorcluster)  [unwired: 1 in]
          }
          frame Error {
            n289 = Format Into String(format string="UI: Update Status >> %s Failed!\nUI: Cursor Set >> Idle\nClose Equipment Resources", error in=w844, w840) -> (resulting string=w841:string, error out=w843:errorcluster)  [unwired: 1 in]
          }
        }
        n290 = Bundle By Name(cluster=w832, "Input Path Loss"=w827, "Path Loss"=w811) -> (w828:T5)
        n291 = call <vilib>:"Add State(s) to Queue__JKI_lib_State_Machine.vi"("State(s) in Front (\"\")"=w822, "State(s) in (\"\")"=w824) -> ("States Out"=w823:string)  [unwired: 13 in]
      }
      frame "Save Calibration" {
        # "// save calibration table to CSV"
        n292 = call "File Dialog"("start path"=path "C:/NGC_TEST/Cal", "default name"="siggen-pwrmeter.cal", "error in"=w968, "pattern (all files)"="*.cal", "pattern label"="Calibration File") -> ("selected path"=w972:path, "cancelled"=w970:bool, "error out"=w971:errorcluster)  [unwired: 7 in, 1 out]
        n293 = Unbundle By Name(w960) -> ("Cal Freqs"=w967:dbl[], "Input Path Loss"=w966:dbl[])
        n294 = control-ref of="Path Loss"() -> (w959:refnum<vi>)
        n295 = case shown="False" w970 {
          tunnel: w966 -> [w985 _]
          tunnel: w967 -> [w991 _]
          tunnel: w971 -> [w983 w997]
          tunnel: [w986 w997] -> w965
          tunnel: w972 -> [w989 _]
          tunnel: w959 -> [w988 _]
          tunnel: "Export Plots to Excel?" -> [w984 _]
          frame False {
            n296 = Build Array(w991, w985) -> (w990:dbl[][])
            n297 = call-poly <vilib>:"Write To Spreadsheet File.vi"("delimiter (\\t)"="," ("delimiter (\\t)"), "transpose? (no:F)"=TRUE, "2D data"=w990, "file path (dialog if empty)"=w989) -> ("new file path (Not A Path if cancelled)"=w987:path)  [unwired: 4 in]
            n298 = case shown="False" w984 {
              tunnel: w988 -> [_ w996]
              tunnel: w987 -> [_ _]
              tunnel: [w993 w995] -> w986
              tunnel: w983 -> [w993 w994]
              frame False {
              }
              frame True {
                n299 = invoke class="WFGraph (strict)" method="Export Data to Excel"(reference=w996, error in=w994) -> (error out=w995:errorcluster)  [unwired: 1 in, 2 out]
              }
            }
          }
          frame True {
          }
        }
        n300 = case shown="No Error" w965 {
          selector: w965 -> [w979 w980]
          tunnel: [w979 w980] -> w964
          tunnel: [w976 "Close Equipment Resources"] -> w961
          tunnel: w957 -> [w977 _]
          frame No Error {
            n301 = Format Into String(format string="UI: Update Status >> %s completed\nClose Equipment Resources\nStop", w977) -> (resulting string=w976:string)  [unwired: 2 in, 1 out]
          }
          frame Error {
          }
        }
        n302 = call <vilib>:"Add State(s) to Queue__JKI_lib_State_Machine.vi"("State(s) in Front (\"\")"=w961, "State(s) in (\"\")"=w963) -> ("States Out"=w962:string)  [unwired: 13 in]
      }
      frame "Close Equipment Resources" {
        n303 = Unbundle By Name(w1005) -> ("PM Type"=w1002:T1, "PSA E4440A GPIB"=w1000:refnum<visa-resource-name>, "U2000 GPIB ALIAS"=w1001:refnum<visa-resource-name>, "EPM GPIB ALIAS"=w999:refnum<visa-resource-name>, "SigGen (ESG)"=w1004:refnum<visa-resource-name>)
        n304 = call "E443X_ESG_VSG_Enable_RF_Output.vi"("VISA Resource Name"=w1004, "Status (T:ON)"=FALSE ("Enable RF Output (F:Disable)"), "error in (no error)"=w1007) -> ("VISA Resource Name Out"=w1011:refnum<visa-resource-name>, "error out"=w1009:errorcluster)  [unwired: 11 in]
        n305 = VISA Close(VISA resource name=w1011, error in (no error)=w1009) -> (error out=w1008:errorcluster)
        n306 = case shown="\"PSA-E444x [E4440]\"" w1002 {
          tunnel: w1008 -> [w1014 w1017 w1020]
          tunnel: [w1013 w1016 w1019] -> w1003
          tunnel: w1001 -> [w1012 _ _]
          tunnel: w1000 -> [_ _ w1018]
          tunnel: w999 -> [_ w1015 _]
          frame "U2000 USB [PM2]" {
            n307 = VISA Close(VISA resource name=w1012, error in (no error)=w1014) -> (error out=w1013:errorcluster)
          }
          frame "E44xx EPM [PM1]" {
            n308 = VISA Close(VISA resource name=w1015, error in (no error)=w1017) -> (error out=w1016:errorcluster)
          }
          frame "PSA-E444x [E4440]" {
            n309 = VISA Close(VISA resource name=w1018, error in (no error)=w1020) -> (error out=w1019:errorcluster)
          }
        }
      }
    }
  }
  "Error Out" <- w11
